vi "Troubleshoot_Apr5_2016.vi"() -> ()   [LabVIEW 2015]
uses:
  <vilib>/Platform/TimedLoop/XDataNode/timing_clust.ctl
  <vilib>/Platform/TimedLoop/XDataNode/nitl_modes.ctl
  <vilib>/Platform/TimedLoop/XDataNode/wakeup.ctl
  <vilib>/FPGAPlugInAG/myRIO-1950/niLvFpga_Open_myRIO-1950.vi
  <vilib>/rvi/interface/common/dynamic/niFpgaDynamicAddResources.vi
  <vilib>/Analysis/3filter.llb/Butterworth Filter (DBL).vi
  <vilib>/Utility/error.llb/Error Cluster From Error Code.vi
  <vilib>/rvi/errors/niLvFpgaAdjustHostInterfaceError.vi
  <vilib>/RVI Host/nirviSupport.llb/nirviErrorClusterFromErrorCode.vi
  <vilib>/rvi/interface/nirviOpenFPGA/nirviOpenFPGA.xnode
  FPGA Bitfiles/Flylaserbox_FPGATarget_FPGAsingleloop_H8b3XToqd60.lvbitx
  FPGA_single_loop.vi
  <vilib>/Platform/TimedLoop/XDataNode/XDataNode.xnode
  <vilib>/rvi/interface/nirviReadWriteControl/nirviReadWriteControl.xnode
  <vilib>/rvi/interface/nirviMethod/nirviMethod.xnode
  <vilib>/Platform/TimedLoop/XDataNode/XDNodeRunTimeDep.lvlib
  <vilib>/rvi/interface/nirviMethod/StockFPGA_InlinedMethodWaitForSingleIRQ.vi
  <vilib>/FPGAPlugInAG/Dynamic/niLvFpga_WaitOnIrq_Dynamic.vi
  NiFpgaLv.dll
  <vilib>/rvi/interface/Simulation/niFpgaSimulationCallBeginRW.vi
  <vilib>/FPGAPlugInAG/Dynamic/niLvFpga_ReadFifo_Dynamic.vi
  <vilib>/rvi/errors/niLvFpgaMergeErrorWithErrorCode.vi
  <vilib>/FPGAPlugInAG/Dynamic/niLvFpga_AcknowledgeIrq_Dynamic.vi
  <vilib>/Analysis/NI_AALBase.lvlib
panel:
  in  "Period":i64
  out "Host loop time":u32=20
  out "Iteration Duration":dbl=4.0 format="%#_6f"
  out "IRQ(s) Asserted":i32
  out "Sensor Loop Time":u32=11
  out "LED loop time":u32=4000
  out "Frame Count":i16=6319
  in  "FPGA Stop":bool
  out "Elements Remaining":u32=3080
  in  "FIFO Timeout setting (ms)":i32=5000
  out "J1":u16[](graph)=[299, 303, 314, 315, 325, 328, 342, 332, 348, 346, 357, 352, 368, 366, 378, 374, 387, 387, 399, 398, 406, 407, 416, 411, 423, 417, 428, 424, 435, 427, 440, 431, 443, 431, 443, 436, 451, 442, 450, 442, 450, 445, 452, 447, 464, 448, 456, 448, 459, 450, 461, 454, 461, 453, 464, 456, 465, 454, 465, 463, 467, 457, 468, 460, 469, 460, 470, 462, 472, 459, 476, 459, 471, 461, 473, 460, 472, 466, 477, 466, 474, 463, 476, 468, 477, 470, 478, 469, 479, 470, 481, 471, 484, 472, 481, 471, 481, 473, 484, 473, 485, 476, 489, 478, 485, 478, 489, 478, 491, 480, 490, 481, 493, 484, 496, 487, 499, 487, 499, 492, 504, 492, 505, 496, 509, 500, 509, 478, 510, 513, 517, 519, 518, 517, 518, 516, 517, 518, 516, 512, 517, 521, 520, 520, 519, 517, 518, 521, 518, 518, 521, 524, 523, 523, 523, 519, 522, 524, 519, 519, 514, 522, 520, 520, 521, 522, 519, 521, 520, 520, 524, 523, 521, 520, 521, 524, 521, 522, 525, 523, 523, 526, 529, 527, 528, 528, 529, 527, 528, 529, 525, 531, 530, 534, 537, 534, 532, 535, 535, 541, 539, 543, 540, 543, 543, 540, 541, 540, 546, 545, 548, 552, 548, 550, 553, 548, 550, 551, 551, 555, 555, 554, 553, 556, 557, 559, 560, 559, 561, 560, 563, 564, 567, 571, 569, 571, 576, 574, 576, 582, 583, 580, 582, 582, 587, 588, 589, 585, 589, 593, 599, 595, 593, 595, 599, 573, 559, 556, 572, 564, 570, 566, 568, 565, 570, 563, 568, 567, 570, 570, 567, 560, 568, 563, 563, 564, 566, 563, 569, 564, 568, 562, 576, 570, 574, 577, 573, 579, 582, 577, 586, 585, 590, 588, 590, 589, 587, 589, 588, 591, 590, 587, 588, 592, 593, 587, 588, 580, 578, 579, 580, 579, 581, 576, 576, 577, 587, 585, 586, 587, 592, 594, 602, 604, 607, 601, 608, 612, 609, 609, 611, 608, 608, 604, 610, 605, 609, 612, 613, 607, 611, 614, 615, 612, 619, 614, 609, 615, 605, 607, 613, 612, 618, 618, 616, 616, 622, 620, 623, 623, 615, 621, 626, 618, 622, 621, 623, 624, 623, 617, 619, 625, 620, 612, 627, 620, 620, 622, 625, 629, 635, 621, 617, 595, 620, 620, 634, 620, 632, 616, 636, 625, 631, 622, 629, 622, 630, 617, 627, 625, 626, 620, 632, 622, 626, 618, 624, 621, 623, 617, 630, 620, 627, 618, 626, 617, 627, 618, 630, 620, 627, 619, 627, 618, 626, 612, 627, 614, 624, 612, 621, 612, 622, 610, 619, 610, 613, 603, 615, 606, 612, 604, 616, 601, 614, 601, 611, 599, 608, 599, 603, 595, 601, 595, 599, 591, 597, 586, 595, 586, 595, 581, 589, 580, 591, 577, 589, 576, 585, 576, 584, 573, 584, 573, 582, 573, 582, 573, 580, 572, 581, 568, 578, 567, 578, 569, 576, 564, 575, 562, 571, 568, 572, 561, 573, 560, 568, 560, 567, 558, 564, 559, 566, 557, 565, 557, 563, 556, 567, 553, 558, 544, 543, 535, 544, 538, 547, 534, 539, 534, 538, 530, 535, 528, 536, 524, 533, 525, 530, 520, 530, 522, 528, 517, 529, 516, 525, 517, 523, 512, 520, 516, 520, 513, 518, 510, 517, 509, 516, 506, 515, 511, 517, 507, 513, 505, 514, 506, 515, 505, 511, 506, 513, 507, 515, 507, 515, 508, 518, 509, 517, 506, 518, 513, 521, 512, 524, 517, 523, 517, 522, 517, 527, 517, 530, 527, 533, 525, 532, 527, 538, 532, 539, 530, 542, 537, 540, 529, 538, 537, 548, 537, 549, 540, 550, 539, 550, 545, 552, 543, 552, 552, 549, 539, 545, 544, 552, 543, 551, 545, 550, 547, 548, 543, 548, 537, 543, 540, 546, 533, 538, 533, 539, 531, 540, 530, 536, 526, 531, 528, 510, 509, 516, 513, 513, 513, 512, 504, 509, 499, 506, 499, 507, 493, 507, 502, 501, 492, 498, 493, 502, 489, 495, 486, 493, 491, 496, 491, 493, 488, 489, 479, 487, 477, 483, 475, 476, 474, 479, 468, 474, 467, 474, 466, 469, 468, 467, 464, 467, 453, 460, 452, 457, 452, 457, 450, 451, 445, 450, 441, 448, 441, 448, 439, 449, 432, 437, 428, 437, 428, 435, 429, 434, 425, 431, 422, 426, 422, 424, 420, 430, 421, 427, 418, 424, 415, 423, 415, 422, 414, 417, 409, 415, 411, 410, 405, 406, 396, 403, 395, 396, 392, 392, 387, 388, 381, 384, 375, 379, 371, 371, 364, 363, 351, 352, 345, 342, 336, 334, 325, 330, 318, 318, 311, 308, 298, 299, 296, 251, 284]
  out "Elements Remaining Real":u32
  out "J4":u16[](graph)=[103, 114, 119, 116, 123, 122, 127, 126, 132, 130, 135, 135, 139, 139, 144, 142, 146, 148, 152, 151, 155, 153, 156, 157, 161, 159, 161, 161, 164, 162, 166, 164, 169, 166, 169, 167, 170, 168, 170, 170, 171, 170, 171, 169, 172, 171, 174, 173, 174, 173, 176, 175, 176, 175, 176, 176, 177, 177, 179, 175, 179, 176, 179, 176, 180, 176, 179, 176, 181, 178, 180, 179, 180, 178, 180, 178, 179, 178, 180, 179, 180, 178, 180, 180, 179, 179, 180, 177, 182, 180, 181, 179, 181, 179, 182, 181, 182, 179, 180, 179, 181, 178, 180, 178, 180, 180, 181, 179, 180, 180, 181, 180, 181, 180, 182, 180, 182, 180, 182, 179, 182, 179, 182, 182, 182, 181, 183, 179, 185, 185, 188, 186, 188, 186, 187, 184, 187, 185, 186, 185, 186, 184, 185, 184, 187, 185, 186, 185, 188, 185, 187, 186, 188, 185, 188, 185, 186, 187, 187, 185, 188, 185, 187, 184, 188, 186, 187, 185, 188, 185, 187, 185, 187, 184, 185, 186, 187, 185, 187, 185, 188, 186, 189, 188, 190, 187, 189, 188, 190, 187, 191, 190, 194, 189, 192, 191, 193, 192, 194, 194, 197, 195, 198, 196, 197, 196, 199, 196, 200, 199, 201, 200, 203, 202, 205, 203, 204, 204, 207, 202, 206, 205, 205, 203, 206, 201, 204, 202, 205, 202, 204, 202, 203, 201, 202, 200, 202, 201, 203, 200, 203, 200, 200, 200, 201, 198, 201, 200, 201, 198, 201, 200, 201, 199, 201, 201, 190, 188, 191, 188, 192, 189, 191, 188, 191, 188, 191, 189, 189, 189, 190, 189, 189, 186, 190, 188, 190, 187, 189, 188, 190, 187, 189, 187, 190, 186, 189, 187, 190, 186, 188, 185, 190, 186, 189, 185, 189, 186, 189, 186, 190, 187, 190, 187, 190, 187, 194, 188, 193, 189, 191, 189, 192, 188, 192, 188, 192, 189, 190, 187, 191, 187, 190, 189, 190, 187, 191, 188, 191, 188, 191, 188, 192, 187, 190, 189, 191, 188, 191, 188, 192, 189, 194, 189, 192, 188, 191, 187, 192, 187, 191, 188, 190, 186, 191, 186, 188, 184, 189, 183, 187, 183, 187, 183, 187, 182, 186, 182, 187, 182, 186, 183, 185, 183, 188, 184, 189, 184, 188, 184, 188, 183, 186, 182, 187, 186, 190, 188, 189, 189, 190, 188, 188, 186, 189, 188, 189, 187, 188, 186, 188, 186, 187, 185, 187, 186, 187, 188, 189, 189, 191, 188, 190, 189, 189, 189, 188, 186, 189, 188, 187, 186, 188, 187, 187, 187, 186, 187, 187, 186, 186, 186, 186, 186, 188, 184, 185, 183, 186, 184, 186, 184, 184, 185, 185, 184, 186, 184, 183, 182, 182, 182, 185, 182, 183, 183, 184, 182, 183, 183, 182, 181, 183, 180, 181, 180, 180, 180, 180, 179, 180, 178, 180, 178, 179, 178, 178, 178, 180, 180, 181, 177, 179, 180, 179, 178, 179, 177, 179, 178, 178, 177, 176, 175, 178, 176, 177, 175, 178, 175, 176, 175, 176, 176, 176, 173, 174, 174, 176, 173, 173, 170, 178, 176, 180, 177, 179, 176, 179, 177, 178, 174, 179, 173, 178, 175, 177, 173, 178, 174, 176, 174, 176, 173, 176, 172, 176, 174, 176, 172, 175, 170, 174, 171, 173, 169, 171, 168, 172, 168, 170, 169, 170, 166, 169, 167, 170, 166, 168, 165, 167, 166, 167, 166, 167, 164, 166, 164, 166, 164, 165, 163, 166, 164, 167, 163, 168, 162, 164, 162, 166, 163, 167, 163, 167, 163, 166, 164, 167, 163, 167, 164, 167, 164, 168, 165, 168, 163, 168, 166, 167, 165, 169, 166, 169, 165, 168, 165, 168, 165, 168, 164, 167, 165, 168, 165, 168, 166, 167, 165, 168, 165, 167, 165, 168, 164, 165, 164, 167, 164, 167, 163, 165, 162, 167, 162, 165, 162, 166, 163, 173, 166, 170, 167, 171, 167, 172, 169, 171, 167, 172, 168, 173, 170, 173, 168, 172, 170, 173, 170, 172, 171, 174, 170, 175, 171, 175, 171, 173, 172, 174, 172, 175, 170, 175, 172, 176, 172, 176, 172, 176, 170, 174, 172, 174, 171, 174, 171, 175, 171, 173, 171, 175, 172, 174, 171, 173, 170, 175, 171, 175, 172, 175, 172, 175, 172, 174, 171, 175, 170, 175, 171, 175, 171, 176, 171, 173, 173, 172, 170, 173, 171, 173, 169, 173, 171, 173, 169, 172, 168, 171, 168, 170, 166, 170, 165, 168, 164, 166, 161, 164, 160, 162, 158, 159, 156, 156, 153, 155, 152, 152, 148, 148, 144, 145, 139, 141, 136, 137, 132, 133, 127, 128, 122, 124, 118, 120, 115, 28, 119]
  out "J8":u16[](graph)=[148, 165, 179, 176, 192, 190, 205, 200, 215, 212, 228, 224, 240, 236, 249, 243, 258, 256, 266, 263, 273, 268, 282, 276, 288, 282, 293, 287, 299, 289, 302, 295, 305, 298, 306, 300, 308, 302, 313, 302, 310, 304, 314, 305, 312, 306, 315, 306, 314, 305, 315, 305, 315, 304, 313, 303, 315, 305, 315, 304, 316, 307, 315, 306, 318, 308, 318, 308, 318, 310, 318, 309, 320, 311, 320, 313, 323, 316, 323, 314, 326, 316, 326, 317, 329, 321, 330, 319, 329, 321, 330, 321, 329, 319, 329, 320, 329, 319, 327, 320, 329, 318, 328, 320, 328, 320, 328, 318, 327, 319, 327, 317, 328, 318, 327, 317, 323, 315, 326, 316, 327, 317, 329, 321, 329, 320, 326, 319, 321, 320, 327, 324, 330, 324, 330, 328, 335, 329, 336, 333, 339, 336, 339, 337, 343, 336, 344, 339, 346, 340, 346, 344, 350, 345, 351, 348, 354, 348, 355, 351, 356, 351, 359, 352, 359, 354, 360, 357, 363, 359, 364, 359, 367, 362, 367, 363, 369, 362, 369, 361, 368, 362, 367, 362, 367, 360, 365, 358, 365, 359, 363, 359, 365, 358, 365, 360, 366, 358, 367, 362, 368, 360, 369, 364, 368, 365, 372, 368, 373, 369, 377, 373, 378, 372, 380, 376, 382, 376, 384, 381, 385, 379, 387, 384, 388, 382, 390, 382, 390, 385, 390, 386, 391, 387, 392, 386, 393, 388, 395, 388, 396, 389, 396, 392, 396, 393, 398, 392, 400, 390, 397, 393, 400, 392, 392, 386, 407, 408, 410, 409, 409, 405, 409, 408, 409, 405, 410, 408, 411, 409, 412, 408, 410, 411, 413, 411, 415, 414, 416, 413, 418, 416, 418, 414, 416, 414, 415, 411, 413, 412, 414, 410, 412, 411, 414, 409, 410, 408, 411, 405, 410, 405, 407, 405, 404, 402, 405, 401, 402, 398, 401, 398, 399, 394, 398, 393, 394, 390, 392, 390, 392, 388, 392, 389, 389, 388, 391, 388, 389, 388, 390, 387, 388, 384, 390, 388, 388, 386, 389, 385, 388, 385, 387, 383, 389, 386, 389, 386, 391, 390, 389, 391, 392, 391, 394, 392, 397, 394, 396, 396, 398, 396, 401, 399, 402, 401, 404, 402, 405, 402, 406, 402, 406, 405, 407, 406, 409, 407, 409, 407, 408, 409, 413, 404, 400, 402, 403, 401, 396, 396, 393, 393, 390, 390, 390, 389, 385, 387, 387, 388, 387, 387, 387, 387, 386, 388, 385, 387, 385, 387, 387, 386, 385, 388, 385, 386, 385, 384, 386, 388, 387, 387, 386, 389, 389, 387, 387, 390, 390, 391, 392, 394, 394, 394, 393, 395, 394, 395, 394, 397, 396, 398, 396, 398, 398, 395, 396, 398, 398, 398, 397, 396, 395, 395, 393, 395, 393, 395, 391, 393, 393, 393, 391, 390, 390, 390, 387, 387, 385, 385, 382, 382, 381, 380, 379, 380, 378, 379, 376, 377, 376, 376, 374, 373, 375, 375, 373, 373, 373, 371, 372, 373, 369, 369, 371, 371, 368, 370, 369, 370, 369, 369, 369, 369, 368, 369, 369, 370, 368, 370, 372, 375, 350, 349, 354, 350, 354, 352, 353, 352, 355, 353, 356, 354, 357, 353, 357, 354, 358, 353, 358, 355, 358, 355, 357, 353, 358, 354, 356, 354, 359, 353, 357, 355, 357, 353, 357, 354, 358, 353, 358, 356, 359, 354, 358, 356, 359, 356, 358, 355, 359, 357, 361, 355, 360, 356, 358, 356, 360, 356, 360, 356, 359, 358, 361, 358, 361, 361, 363, 360, 365, 363, 368, 363, 365, 363, 367, 363, 367, 363, 366, 363, 366, 363, 367, 361, 362, 359, 359, 356, 357, 353, 355, 351, 354, 351, 355, 350, 353, 349, 353, 352, 353, 349, 352, 348, 351, 346, 350, 346, 347, 342, 348, 344, 346, 341, 348, 344, 345, 342, 345, 341, 345, 342, 342, 338, 342, 337, 337, 333, 334, 342, 335, 340, 337, 341, 337, 342, 339, 341, 335, 339, 335, 340, 334, 339, 334, 339, 331, 336, 332, 334, 331, 336, 330, 335, 331, 335, 326, 334, 329, 333, 328, 333, 328, 333, 327, 334, 328, 333, 328, 334, 329, 333, 328, 332, 327, 331, 324, 330, 327, 331, 326, 331, 325, 329, 324, 330, 326, 327, 326, 329, 325, 330, 325, 329, 325, 329, 325, 330, 323, 329, 325, 327, 323, 328, 325, 325, 321, 324, 318, 324, 317, 322, 318, 315, 303, 309, 310, 312, 309, 311, 306, 309, 304, 305, 301, 301, 297, 298, 293, 293, 285, 286, 281, 283, 276, 275, 269, 271, 262, 261, 254, 253, 244, 243, 236, 233, 226, 220, 214, 211, 202, 200, 193, 189, 180, 178, 125, 198]
  out "J5":u16[](graph)=[173, 183, 200, 196, 214, 209, 228, 224, 240, 234, 253, 246, 263, 257, 274, 266, 284, 278, 291, 283, 299, 289, 307, 296, 312, 302, 318, 307, 320, 309, 323, 312, 324, 313, 324, 315, 326, 315, 327, 319, 329, 318, 331, 318, 332, 321, 334, 323, 338, 324, 338, 327, 339, 327, 340, 328, 344, 331, 343, 332, 345, 334, 347, 336, 350, 339, 351, 339, 352, 340, 354, 343, 357, 345, 359, 348, 360, 350, 363, 351, 364, 352, 365, 354, 367, 355, 367, 358, 370, 358, 371, 358, 369, 359, 371, 361, 373, 360, 372, 360, 371, 359, 372, 360, 372, 360, 371, 359, 371, 359, 369, 358, 371, 358, 369, 354, 367, 357, 367, 354, 368, 354, 367, 354, 364, 353, 362, 342, 355, 345, 350, 344, 349, 344, 347, 344, 348, 340, 347, 340, 346, 341, 348, 341, 346, 339, 345, 339, 345, 338, 343, 337, 344, 338, 342, 338, 341, 338, 344, 339, 344, 338, 342, 339, 344, 339, 344, 340, 346, 340, 347, 341, 347, 343, 349, 344, 350, 346, 352, 347, 353, 350, 357, 352, 357, 353, 360, 358, 364, 360, 367, 364, 373, 367, 372, 372, 379, 375, 380, 378, 386, 384, 391, 387, 394, 392, 399, 397, 406, 401, 409, 405, 412, 408, 415, 412, 419, 417, 424, 420, 426, 421, 428, 426, 432, 429, 435, 431, 438, 434, 440, 438, 442, 441, 446, 441, 449, 444, 453, 450, 457, 455, 461, 457, 463, 463, 469, 466, 474, 468, 475, 472, 478, 474, 479, 471, 476, 462, 464, 462, 465, 463, 465, 462, 468, 461, 465, 461, 463, 459, 463, 459, 461, 457, 458, 454, 457, 452, 453, 451, 452, 446, 448, 444, 448, 442, 445, 440, 444, 437, 441, 436, 439, 436, 439, 435, 439, 434, 438, 436, 439, 435, 438, 435, 440, 436, 441, 440, 444, 440, 445, 444, 447, 445, 451, 448, 449, 446, 451, 448, 454, 449, 456, 452, 455, 454, 459, 457, 460, 458, 463, 460, 462, 458, 463, 460, 465, 464, 468, 463, 468, 466, 468, 466, 468, 465, 471, 468, 469, 464, 466, 464, 467, 462, 466, 462, 464, 461, 462, 459, 460, 457, 459, 459, 460, 454, 456, 452, 455, 452, 454, 448, 451, 446, 451, 443, 447, 443, 444, 440, 439, 436, 438, 437, 441, 438, 438, 434, 437, 437, 438, 437, 437, 438, 439, 437, 439, 437, 436, 435, 440, 437, 437, 435, 438, 434, 434, 436, 436, 436, 437, 434, 434, 433, 434, 432, 432, 432, 432, 432, 434, 431, 431, 431, 429, 430, 430, 429, 429, 427, 428, 425, 427, 425, 426, 425, 424, 424, 422, 419, 422, 419, 421, 417, 420, 416, 418, 416, 418, 412, 413, 411, 413, 411, 410, 409, 409, 407, 408, 405, 405, 404, 403, 403, 403, 401, 402, 400, 400, 399, 399, 398, 400, 397, 398, 397, 397, 395, 396, 396, 397, 395, 395, 394, 394, 392, 393, 392, 393, 390, 390, 389, 391, 389, 389, 387, 388, 387, 389, 385, 386, 384, 385, 382, 384, 380, 380, 381, 380, 376, 376, 381, 402, 382, 392, 379, 390, 381, 391, 382, 393, 383, 392, 382, 391, 384, 392, 385, 393, 385, 393, 383, 392, 383, 391, 381, 392, 384, 390, 380, 390, 380, 391, 381, 392, 381, 389, 379, 389, 379, 390, 378, 388, 380, 389, 378, 386, 378, 388, 378, 387, 376, 389, 379, 386, 377, 388, 379, 388, 378, 389, 380, 391, 380, 390, 381, 391, 382, 392, 383, 393, 384, 394, 384, 394, 383, 394, 386, 396, 384, 392, 384, 394, 383, 394, 384, 392, 381, 389, 379, 390, 379, 386, 377, 386, 372, 383, 372, 381, 371, 379, 369, 377, 367, 375, 366, 373, 363, 373, 363, 371, 361, 369, 358, 367, 356, 365, 356, 363, 353, 361, 352, 359, 349, 358, 347, 359, 349, 354, 352, 355, 349, 352, 348, 352, 350, 351, 350, 351, 349, 353, 351, 351, 347, 349, 345, 351, 345, 348, 344, 349, 344, 345, 344, 347, 342, 344, 341, 344, 341, 343, 341, 345, 341, 345, 340, 342, 339, 340, 343, 341, 339, 340, 338, 339, 338, 339, 337, 338, 336, 338, 336, 337, 337, 340, 337, 338, 339, 338, 338, 339, 336, 337, 336, 338, 335, 337, 334, 337, 334, 336, 333, 337, 333, 333, 334, 335, 332, 333, 332, 332, 329, 329, 327, 330, 326, 326, 324, 325, 322, 322, 319, 321, 318, 320, 316, 317, 313, 314, 309, 311, 305, 307, 302, 301, 297, 295, 289, 289, 284, 283, 277, 276, 268, 267, 261, 257, 248, 244, 237, 234, 227, 223, 215, 212, 202, 200, 195, 172, 227]
  out "Finished Late? [i-1]":bool
  out "Has timed loop ever been late?":bool
  in  "Threshold for noise filter":dbl=8.0
  out "Fly real-time location/center mass":dbl(graph)=731.3095378093176
  in  "Fly presence? J1":bool=TRUE
  in  "Threshhold position filter J1":i32=25
  out "Fly real-time location J1":dbl(graph)=731.3095378093176
  in  "Threshold for noise filter J4":dbl=7.0
  in  "Threshhold position filter J4":i32=25
  in  "Fly presence? J4":bool=TRUE
  out "Fly real-time location J4":dbl(graph)=203.38593568844155
  in  "Threshold for noise filter J5":dbl=5.0
  in  "Threshhold position filter J5":i32=25
  out "Fly real-time location J5":dbl(graph)=118.45001929078613
  in  "Fly presence? J5":bool=TRUE
  in  "Threshold for noise filter J8":dbl=5.0
  in  "Threshhold position filter J8":i32=25
  in  "Fly presence? J8":bool=TRUE
  out "Fly real-time location J8":dbl(graph)=209.002598036444
  out "Noise check J1":dbl[](graph)=[0.0, 0.0, 0.0, 0.0, 0.0, 0.0, 0.0, 0.0, 0.0, 0.0, 0.0, 0.0, 0.0, 0.0, 0.0, 0.0, 0.0, 0.0, 0.0, 0.0, 0.0, 0.0, 0.0, 0.0, 0.0, 0.0, 0.0, 0.0, 0.0, 0.0, 0.0, 0.0, 0.0, 0.0, 0.0, 0.0, 0.0, 0.0, 0.0, 0.0, 0.0, 0.0, 0.0, 0.0, 0.0, 0.0, 0.0, 0.0, 0.0, 0.0, 0.0, 0.0, 0.0, 0.0, 0.0, 0.0, 0.0, 0.0, 0.0, 0.0, 0.0, 0.0, 0.0, 0.0, 0.0, 0.0, 0.0, 0.0, 0.0, 0.0, 0.0, 0.0, 0.0, 0.0, 0.0, 0.0, 0.0, 0.0, 0.0, 0.0, 0.0, 0.0, 0.0, 0.0, 0.0, 0.0, 0.0, 0.0, 0.0, 0.0, 0.0, 0.0, 0.0, 0.0, 0.0, 0.0, 0.0, 0.0, 0.0, 0.0, 0.0, 0.0, 0.0, 0.0, 0.0, 0.0, 0.0, 0.0, 0.0, 0.0, 0.0, 0.0, 0.0, 0.0, 0.0, 0.0, 0.0, 0.0, 0.0, 0.0, 0.0, 0.0, 0.0, 0.0, 0.0, 0.0, 0.0, 0.0, 0.0, 0.0, 0.0, 0.0, 0.0, 0.0, 0.0, 0.0, 0.0, 0.0, 0.0, 0.0, 0.0, 0.0, 0.0, 0.0, 0.0, 0.0, 0.0, 0.0, 0.0, 0.0, 0.0, 0.0, 0.0, 0.0, 0.0, 0.0, 0.0, 0.0, 0.0, 0.0, 0.0, 0.0, 0.0, 0.0, 0.0, 0.0, 0.0, 0.0, 0.0, 0.0, 0.0, 0.0, 0.0, 0.0, 0.0, 0.0, 0.0, 0.0, 0.0, 0.0, 0.0, 0.0, 0.0, 0.0, 0.0, 0.0, 0.0, 0.0, 0.0, 0.0, 0.0, 0.0, 0.0, 0.0, 0.0, 0.0, 0.0, 0.0, 0.0, 0.0, 0.0, 0.0, 0.0, 0.0, 0.0, 0.0, 0.0, 0.0, 0.0, 0.0, 0.0, 0.0, 0.0, 0.0, 0.0, 0.0, 0.0, 0.0, 0.0, 0.0, 0.0, 0.0, 0.0, 0.0, 0.0, 0.0, 0.0, 0.0, 0.0, 0.0, 0.0, 0.0, 0.0, 0.0, 0.0, 0.0, 0.0, 0.0, 0.0, 0.0, 0.0, 0.0, 0.0, 0.0, 0.0, 0.0, 0.0, 0.0, 0.0, 0.0, 0.0, 0.0, 0.0, 0.0, 0.0, 0.0, 0.0, 0.0, 0.0, 0.0, 0.0, 0.0, 0.0, 0.0, 0.0, 0.0, 0.0, 0.0, 0.0, 0.0, 0.0, 0.0, 0.0, 0.0, 0.0, 0.0, 0.0, 0.0, 0.0, 0.0, 0.0, 0.0, 0.0, 0.0, 0.0, 0.0, 0.0, 0.0, 0.0, 0.0, 0.0, 0.0, 0.0, 0.0, 0.0, 0.0, 0.0, 0.0, 0.0, 0.0, 0.0, 0.0, 0.0, 0.0, 0.0, 0.0, 0.0, 0.0, 0.0, 0.0, 0.0, 0.0, 0.0, 0.0, 0.0, 0.0, 0.0, 0.0, 0.0, 0.0, 0.0, 0.0, 0.0, 0.0, 0.0, 0.0, 0.0, 0.0, 0.0, 0.0, 0.0, 0.0, 0.0, 0.0, 0.0, 0.0, 0.0, 0.0, 0.0, 0.0, 0.0, 0.0, 0.0, 0.0, 0.0, 0.0, 0.0, 0.0, 0.0, 0.0, 0.0, 0.0, 0.0, 0.0, 0.0, 0.0, 0.0, 0.0, 0.0, 0.0, 0.0, 0.0, 0.0, 0.0, 0.0, 0.0, 0.0, 0.0, 0.0, 0.0, 0.0, 0.0, 0.0, 0.0, 0.0, 0.0, 0.0, 0.0, 0.0, 0.0, 0.0, 0.0, 0.0, 0.0, 0.0, 0.0, 0.0, 0.0, 0.0, 0.0, 0.0, 0.0, 0.0, 0.0, 0.0, 0.0, 0.0, 0.0, 0.0, 0.0, 0.0, 0.0, 0.0, 0.0, 0.0, 0.0, 0.0, 0.0, 0.0, 0.0, 0.0, 0.0, 0.0, 0.0, 0.0, 0.0, 0.0, 0.0, 0.0, 0.0, 0.0, 0.0, 0.0, 0.0, 0.0, 0.0, 0.0, 0.0, 0.0, 0.0, 0.0, 0.0, 0.0, 0.0, 0.0, 0.0, 0.0, 0.0, 0.0, 0.0, 0.0, 0.0, 0.0, 0.0, 0.0, 0.0, 0.0, 0.0, 0.0, 0.0, 0.0, 0.0, 0.0, 0.0, 0.0, 0.0, 0.0, 0.0, 0.0, 0.0, 0.0, 0.0, 0.0, 0.0, 0.0, 0.0, 0.0, 0.0, 0.0, 0.0, 0.0, 0.0, 0.0, 0.0, 0.0, 0.0, 0.0, 0.0, 0.0, 0.0, 0.0, 0.0, 0.0, 0.0, 0.0, 0.0, 0.0, 0.0, 0.0, 0.0, 0.0, 0.0, 0.0, 0.0, 0.0, 0.0, 0.0, 0.0, 0.0, 0.0, 0.0, 0.0, 0.0, 0.0, 0.0, 0.0, 0.0, 0.0, 0.0, 0.0, 0.0, 0.0, 0.0, 0.0, 0.0, 0.0, 0.0, 0.0, 0.0, 0.0, 0.0, 0.0, 0.0, 0.0, 0.0, 0.0, 0.0, 0.0, 0.0, 0.0, 0.0, 0.0, 0.0, 0.0, 0.0, 0.0, 0.0, 0.0, 0.0, 0.0, 0.0, 0.0, 0.0, 0.0, 0.0, 0.0, 0.0, 0.0, 0.0, 0.0, 0.0, 0.0, 0.0, 0.0, 0.0, 0.0, 0.0, 0.0, 0.0, 0.0, 0.0, 0.0, 0.0, 0.0, 0.0, 0.0, 0.0, 0.0, 0.0, 0.0, 0.0, 0.0, 0.0, 0.0, 0.0, 0.0, 0.0, 0.0, 0.0, 0.0, 0.0, 0.0, 0.0, 0.0, 0.0, 0.0, 0.0, 0.0, 0.0, 0.0, 0.0, 0.0, 0.0, 0.0, 0.0, 0.0, 0.0, 0.0, 0.0, 0.0, 0.0, 0.0, 0.0, 0.0, 0.0, 0.0, 0.0, 0.0, 0.0, 0.0, 0.0, 0.0, 0.0, 0.0, 0.0, 0.0, 0.0, 0.0, 0.0, 0.0, 0.0, 0.0, 0.0, 0.0, 0.0, 0.0, 0.0, 0.0, 0.0, 0.0, 0.0, 0.0, 0.0, 0.0, 0.0, 0.0, 0.0, 0.0, 0.0, 0.0, 0.0, 0.0, 0.0, 0.0, 0.0, 0.0, 0.0, 0.0, 0.0, 0.0, 0.0, 0.0, 0.0, 0.0, 0.0, 0.0, 0.0, 0.0, 0.0, 0.0, 0.0, 0.0, 0.0, 0.0, 0.0, 0.0, 0.0, 0.0, 0.0, 0.0, 0.0, 0.0, 0.0, 0.0, 0.0, 0.0, 0.0, 0.0, 0.0, 0.0, 0.0, 0.0, 0.0, 0.0, 0.0, 0.0, 0.0, 0.0, 0.0, 0.0, 0.0, 0.0, 0.0, 0.0, 0.0, 0.0, 0.0, 0.0, 0.0, 0.0, 0.0, 0.0, 0.0, 0.0, 0.0, 0.0, 0.0, 0.0, 0.0, 0.0, 0.0, 0.0, 0.0, 0.002630031854768592, 0.02647244479643197, 0.07238343896731143, 0.0945645708112122, 0.07323461692650168, 0.0403804808476501, 0.05121951335433386, 0.1762106489274184, 0.44006181658327786, 0.7845113623785474, 1.119997669332286, 1.3668328869065776, 1.4775687137089684, 1.4816747529196042, 1.4845963350311595, 1.5954761742667545, 1.8331785662226308, 2.090278012312389, 2.2184400479496444, 2.1448325104345916, 1.9046852618093164, 1.611675881479425, 1.3951054047298297, 1.310250193006133, 1.3163036215716177, 1.3380381305237252, 1.2993463614109941, 1.1409959811952943, 0.8726900095644392, 0.5720582464254442, 0.3083972063095004, 0.1147690458320547, 0.00540622533437389, -0.033159310484607185, -0.033064972848972515, -0.02012085186680765, -0.007948463448035415, -0.0007869325832231132, 0.0019075606614335245, 0.002060776300040158, 0.0013070649745447168, 0.0005453872425892686, 7.850769862843349e-05, -0.00010777797942906934, -0.00012778328636531668, -8.45492446052674e-05, -3.7119363484340684e-05, -6.8133899757183335e-06, 5.949395488515054e-06, 7.88027385042564e-06, 5.4464616068189726e-06, 2.508215297396619e-06, 5.492808583469846e-07, -3.1820480618137934e-07, -4.830999877916673e-07]
  out "Noise check J4":dbl[](graph)
  out "Noise check J5":dbl[](graph)=[0.0, 0.0, 0.0, 0.0, 0.0, 0.0, 0.0, 0.0, 0.0, 0.0, 0.0, 0.0, 0.0, 0.0, 0.0, 0.0, 0.0, 0.0, 0.0, 0.0, 0.0, 0.0, 0.0, 0.0, 0.0, 0.0, 0.0, 0.0, 0.0, 0.0, 0.0, 0.0, 0.0, 0.0, 0.0, 0.0, 0.0, 0.0, 0.0, 0.0, 0.0, 0.0, 0.0, 0.0, 0.0, 0.0, 0.0, 0.0, 0.0, 0.0, 0.0, 0.0, 0.0, 0.0, 0.0, 0.0, 0.0, 0.0, 0.0, 0.0, 0.0, 0.0, 0.0, 0.0, 0.0, 0.0, 0.0, 0.0, 0.0, 0.0, 0.0, 0.0, 0.0, 0.0, 0.0, 0.0, 0.0, 0.0, 0.012054538365298214, 0.08251007933289906, 0.2697925233234689, 0.5818524655936519, 0.9729636503034512, 1.3844748873925616, 1.7368973639426482, 1.9514883967448342, 2.049795713035472, 2.147680935919143, 2.3188998494047826, 2.5331530921105125, 2.708069472184627, 2.8118388391573657, 2.9368447973981366, 3.211657108218735, 3.6431393080511585, 4.115369018049598, 4.513477004341131, 4.788356388610584, 4.94484597379937, 5.027249271232393, 5.089663667941105, 5.167005021431631, 5.29495778292663, 5.524154011291435, 5.879990611460722, 6.317736798856551, 6.728055846578749, 6.994230662169988, 7.050570723594823, 6.91770548084906, 6.7126808158556095, 6.591977061099051, 6.647863503971012, 6.837387129399459, 7.006122980790215, 7.02845268511157, 6.943869825354531, 6.8908804792545695, 6.913056904386163, 6.940669455926634, 6.926706265783624, 6.891548364808854, 6.879976507396142, 6.9238783794600405, 7.014599560394951, 7.097802219395696, 7.099555418502421, 6.98268555249647, 6.792270609676624, 6.6049691690102215, 6.434305425951933, 6.237108330326169, 6.01320772445422, 5.836092870646612, 5.7530536936199, 5.715991836295783, 5.633548975996455, 5.4546187281227265, 5.208524422197506, 4.96463488228587, 4.769010412200817, 4.626611813331992, 4.494516771543445, 4.31103555561957, 4.054161846296417, 3.746066456881264, 3.4211563867039594, 3.099985192886244, 2.7794014976662895, 2.44637263169793, 2.0912750035506713, 1.7110175602290862, 1.3259640476500372, 0.9785330169390857, 0.6675468418740619, 0.3718185768752308, 0.13600990134847535, 0.00429183911095006, -0.04129024906400588, -0.04035943318370341, -0.024287822164054097, -0.009445633942039625, -0.0008094883626780184, 0.0023853516999582454, 0.002518760604299784, 0.0015795930379951223, 0.0006496677301419525, 8.598159733688785e-05, -0.0001354916826684314, -0.0001564033159245941, -0.00010229456616431273, -4.430980324289726e-05, -7.677494406688178e-06, 7.531523270977754e-06, 9.659953038992932e-06, 6.5969833094280795e-06, 2.9997111649637766e-06, 6.291603719864854e-07, -4.067256343405995e-07, -5.931847294950123e-07, -4.2368471484944137e-07, -2.017255367751674e-07, -4.896042170647565e-08, 2.108151732718652e-08, 3.6195985715165595e-08, 2.709873015883781e-08, 1.3483599237422958e-08, 3.6795492211654384e-09, -1.025420804479972e-09, -2.1932924129452164e-09, -1.7260489829314328e-09, -8.962371163395401e-10, -2.696307957092095e-10, 4.4535353362904505e-11, 1.3186526572366835e-10, 1.0947864700726096e-10, 5.92623696840606e-11, 1.9380215627957422e-11, -1.4822807061719387e-12, -7.857579527927355e-12, -6.914103455156049e-12, -3.89948607597912e-12, -1.371769578237791e-12, 6.511930663237629e-15, 4.633960331867196e-13, 4.347233263672884e-13, 2.553957382901364e-13, 9.58816357857041e-14, 5.266160377061325e-15, -2.6995561643986745e-14, -2.720704639289042e-14, -1.665252878596416e-14, -6.631139240315776e-15, -7.0105510310460695e-16, 1.5494186569176565e-15, 1.6944909533061055e-15, 1.0811085060167869e-15, 4.54448556635201e-16, 6.808870612399017e-17, -8.728820444841173e-17, -1.0499234375208962e-16, -6.989166283689154e-17, -3.0897043736463205e-17, -5.832791247263445e-18, 4.7998062532403726e-18, 6.469564482484962e-18, 4.499628471438213e-18, 2.0857689124703708e-18, 4.666056321817816e-19, -2.5533629528269204e-19, -3.9626857856385e-19, -2.8849350033730597e-19, -1.3990475436771997e-19, -3.573896726576872e-20, 1.293989664760119e-20, 2.4112840645085403e-20, 1.8420505295880255e-20, 9.329405395104378e-21, 2.655679327128802e-21, -6.06003317208522e-22, -1.456571849069185e-21, -1.1712680032801579e-21, -6.187581139185739e-22, -1.9294807659464302e-22, 2.433951347022674e-23, 8.726353889898586e-23, 7.415968231766969e-23, 4.0830572710290474e-23, 1.377553901834581e-23, -6.2248816426723375e-25, -5.178733808997571e-24, -4.675061004313882e-24, -2.681445181815658e-24, -9.697370938178341e-25, -2.046183940374795e-26, 3.0395409074202434e-25, 2.93391278112018e-25, 1.7529391947798681e-25, 6.747159951419807e-26, 5.181527579327607e-27, -1.7605342120402465e-26, -1.8325651591036842e-26, -1.1409142639444767e-26, -4.648092306822356e-27, -5.792159064985569e-28, 1.0032741085991282e-27, 1.138967869605295e-27, 7.394045026689562e-28, 3.1746129396768222e-28, 5.283721074875335e-29, -5.600503129665911e-29, -7.04144534634944e-29, -4.7719039617888896e-29, -2.1518457519526855e-29, -4.381449771013153e-30, 3.041948713826757e-30, 4.328460008429178e-30, 3.066928327464483e-30, 1.4487077542079428e-30, 3.435453267891325e-31, -1.590049444459223e-31, -2.6442640820958e-31, -1.963019603444207e-31, -9.693312702314344e-32, -2.5955441804768686e-32, 7.840017129254836e-33, 1.6043452970542605e-32, 1.251257347573923e-32, 6.449149749539311e-33, 1.9094588691359505e-33, -3.4946149682933526e-34, -9.659617486074822e-34, -7.942303047997757e-34, -4.268202629278789e-34, -1.3766656808557905e-34, 1.2480135861303e-35, 5.765524095873537e-35, 5.01978371833872e-35, 2.8108561111449943e-35, 9.768393167274569e-36, -1.5979097064840415e-37, -3.406783427648679e-36, -3.158682561416305e-36, -1.8424400025079897e-36, -6.8417490579824315e-37, -3.08996197074768e-38, 1.9892586109109132e-37, 1.97848973677004e-37, 1.2022518088671383e-37, 4.739972967349818e-38, 4.6138334091484117e-39, -1.1449946036667541e-38, -1.2333057118713003e-38, -7.811069082981466e-39, -3.253327516286039e-39, -4.6357690325503895e-40, 6.473780095712158e-40, 7.648794751634878e-40, 5.053426150476074e-40, 2.2148176150911223e-40, 4.0367468947110693e-41, -3.576843912725162e-41, -4.717863079482069e-41, -3.25576266404017e-41, -1.496941450408354e-41, -3.260757128172403e-42, 1.9155335318504096e-42, 2.892901376006323e-42, 2.0889423964204834e-42, 1.0051733200205593e-42, 2.5137236233228282e-43, -9.806163732946778e-44, -1.7624418575065763e-43, -1.3347739940883268e-43, -6.709563709262192e-44, -1.8765906832021888e-44, 4.672545729490458e-45, 1.0660620638309889e-44, 8.493414283511421e-45, 4.454127567626845e-45, 1.3682536486147045e-45, -1.947072781173578e-46, -6.396563318091131e-46, -5.3817134709572885e-46, -2.9417403469254757e-46, -9.795949067489972e-47, 5.70091804711327e-48, 3.8028040638436656e-47, 3.395287453186378e-47, 1.9335063550196973e-47, 6.911647890734894e-48, 7.134294021746332e-50, -2.2366198611548918e-48, -2.1324864077513384e-48, -1.2649875125605185e-48, -4.818128617466808e-49, -3.259501821845982e-50, 1.2987340936199763e-49, 1.3331083068039984e-49, 8.239552005229725e-50, 3.3246297731028743e-50, 3.8797367491773775e-51, -7.424248357593614e-51, -8.292894061549167e-51, -5.343866049579547e-51, -2.2739472080306295e-51, -3.6260930461838345e-52, 4.1611107172087994e-52, 5.1318304892697584e-52, 3.451299279413764e-52, 1.5433060027470366e-52, 3.046097601798571e-53, -2.27246498197299e-53, -3.1578663989489454e-53, -2.219776665712926e-53, -1.0402033777440495e-53, -2.4078759438364993e-54, 1.1971773816231694e-54, 1.9313349743840303e-54, 1.4218209489652026e-54, 6.967273214005052e-55, 1.8294050181191415e-55, -5.976448128700266e-56, -1.1732666059348616e-55, -9.069514266383446e-56, -4.639931366654287e-56, -1.351397822674065e-56, 2.725337028933403e-57, 7.074131801150358e-57, 5.761109747156628e-57, 3.073582425449035e-57, 9.774313850422019e-58, -1.0299632780581152e-58, -4.229163307858031e-58, -3.6439723122896195e-58, -2.0258489406820065e-58, -6.95331260724567e-59, 1.9718380721558834e-60, 2.503677545378321e-59, 2.294761891250138e-59, 1.3289630775558111e-59, 4.880377750316307e-60, 1.7138734414810517e-61, -1.4652070457631984e-60, -1.438539565251322e-60, -8.678657602047437e-61, -3.387184971834156e-61, -3.0058274960698244e-62, 8.456695232049919e-62, 8.974991225370526e-62, 5.642804464715705e-62, 2.3284233274234247e-62, 3.1432374415349554e-63, -4.797938411692989e-63, -5.571285529343017e-63, -3.6533455664022435e-63, -1.587312055580106e-63, -2.7875030234571983e-64, 2.6629571313142356e-64, 3.439827735234227e-64, 2.355448313158835e-64, 1.0741287215472925e-64, 2.2754883277815795e-65, -1.4350781023773857e-65, -2.1115007195583554e-65, -1.5123826022475209e-65, -7.220544185442533e-66, -1.766319002352943e-66, 7.415465360776138e-67, 1.287909779752148e-66, 9.670708063997506e-67, 4.824598402063589e-67, 1.3251056408020904e-67, -3.588778881549252e-68, -7.800551980437032e-68, -6.1581713093038186e-68, -3.2057955965438806e-68, -9.697293041175945e-69, 1.543289763721433e-69, 4.687458556742928e-69, 3.9049483880979624e-69, 2.119134461629086e-69, 6.962896680527191e-70, -4.990995927608514e-71, -2.7915211688805858e-70, -2.4655048668680618e-70, -1.3939932242542608e-70, -4.924344601083624e-71, 3.927467080077828e-74, 1.645151051834821e-71, 1.5497541307447514e-71, 9.12738522750362e-72, 3.4395342160104647e-72, 2.0036221518433227e-73, -9.576080972696221e-73, -9.696289774594392e-73, -5.949722678388557e-73, -2.3773557445591164e-73, -2.5815159823120656e-74, 5.49064253941797e-74, 6.037132757695715e-74, 3.861649169380785e-74, 1.6284201664114956e-74, 2.4807286659373073e-75, -3.089213805414149e-75, -3.7394482624370276e-75, -2.495847697215915e-75, -1.10662502120126e-75, -2.113868432241852e-76, 1.6957758000383484e-76, 2.3034155675194953e-76, 1.6064224235654762e-76, 7.467443963645365e-77, 1.6856322745473272e-77, -8.9991863865603e-78, -1.4103288540622355e-77, -1.0296979156619355e-77, -5.006988869635323e-78, -1.2883079918531505e-78, 4.543678668168596e-79, 8.578181303236732e-79, 6.573027336965598e-79, 3.337715836111659e-79, 9.558195561958412e-80, -2.1141662566815895e-80, -5.179320249526578e-80, -4.178387874942195e-80, -2.212981784556838e-80, -6.936232770225309e-81, 8.37062978236571e-82, 3.101268134330151e-81, 2.6448826446712786e-81, 1.4598632265428433e-81, 4.9474470123399654e-82, -2.0171297916052668e-83, -1.8393258246703207e-82, -1.666895358194387e-82, -9.584554068533997e-83, -3.480086374698044e-83, -8.620554337386052e-85, 1.078753425838644e-83, 1.0457936646429192e-83, 6.2639924737503615e-84, 2.41976985851077e-84, 1.9338340990158314e-85, -6.242663254897406e-85, -6.530250726607995e-85, -4.0758916772113865e-85, -1.6660372835813097e-85, -2.1212445550281623e-86, 3.553529066050428e-86, 4.057380851339728e-86, 2.640825663101548e-86, 1.1373340286341773e-86, 1.9201358446140602e-87, -1.980791993412643e-87, -2.507553882420818e-87, -1.7038804747963386e-87, -7.705826232728537e-88, -1.5855210624222498e-88, 1.07376515097235e-88, 1.5408625136798773e-88, 1.0948173927414702e-88, 5.1858289886466615e-89, 1.2398551494562039e-89, -5.596630177228314e-90, -9.409404031669224e-90, -7.005727804547023e-90, -3.4685955064333816e-90, -9.349806035406329e-91, 2.746903354224976e-91, 5.706407330517513e-91, 4.4644179747537506e-91, 2.3069578551601477e-91, 6.868813994758339e-92, -1.2138795779969215e-92, -3.434061306446763e-92, -2.8330375230661456e-92, -1.5263262897390942e-92, -4.946883853483729e-93, 4.237874744095357e-94, 2.048511947077114e-93, 1.7900930940233344e-93, 1.0048786386264384e-93, 3.5071096818190274e-94, -4.3060744249157035e-96, -1.2096346196217003e-94, -1.1261008749736332e-94, -6.584865467847136e-95, -2.454601117442337e-95, -1.1926497105302533e-96, 7.057562794279636e-96, 7.051483917490095e-96, 4.295681862553622e-96, 1.6995130606122677e-96, 1.704223256475097e-97, -4.058286440295077e-97, -4.394263568065116e-97, -2.7901892763014225e-97, -1.1658611547339225e-97, -1.6912134581197252e-98, 2.2917125095525306e-98, 2.7243850940860876e-98, 1.8046707296049194e-98, 7.93331516254654e-99, 1.4640321662858872e-99, -1.264135623974204e-99, -1.679849218164158e-99, -1.1623984900549929e-99, -5.359700669571324e-100, -1.1785126179286392e-100, 6.754545380554396e-101, 1.0296621849658506e-100, 7.456233050757999e-101, 3.5975966531781505e-101, 9.064356356623966e-102, -3.446031714780245e-102, -6.27040197714801e-102, -4.763114440149107e-102, -2.400573367879994e-102, -6.755774628353267e-103, 1.632505823764485e-103, 3.7910661271982855e-103, 3.0300828140365445e-103, 1.5931007647499802e-103, 4.919622004787324e-104, -6.720717752203688e-105, -2.2735093478656468e-104, -1.9194612442156153e-104, -1.0518489667242896e-104, -3.5187230146787246e-105, 1.8867934935230323e-106, 1.3507962680887472e-105, 1.2106498184386113e-105, 6.911461723173569e-106, 2.4806892083610147e-106, 3.499564060662571e-108, -7.939021964071217e-107, -7.601633824400351e-107, -4.5205484457502814e-107, -1.728136006096324e-107, -1.2245276971436868e-108, 4.6059575691196815e-108, 4.750714340357272e-108, 2.943697244355842e-108, 1.1917729308731339e-108, 1.4238187995466512e-109, -2.630187198456678e-109, -2.954370538273902e-109, -1.9086781895160755e-109, -8.147288751216045e-110, -1.3190768673060703e-110, 1.4721253200341085e-110, 1.827625351172069e-110, 1.2323932656982504e-110, 5.527030632944665e-111, 1.102956901513762e-111, -8.024658050923763e-112, -1.1242243171061093e-111, -7.924402492366014e-112, -3.723783928584415e-112, -8.69349659312024e-113, 4.2163059043247584e-113, 6.873003526379965e-113, 5.074494566054847e-113, 2.4932781828755692e-113, 6.59187025309434e-114, -2.0960524006987115e-114, -4.173467239373314e-114, -3.2360985144614554e-114, -1.6598671924267714e-114, -4.86238292024909e-115, 9.485920605775333e-116, 2.5151354782351553e-115, 2.055095116158086e-115, 1.099183764079932e-115, 3.5128868574873646e-116, -3.519643889725524e-117, -1.5027974940673502e-116, -1.2995296020827136e-116, -7.242757606246731e-117, -2.4967720168809652e-117, 6.027330313111894e-119, 8.890835541183572e-118, 8.181449125009961e-118, 4.74993236124186e-118, 1.7511294687454097e-118, 6.766990903334703e-120, -5.199100208354612e-119, -5.127325047972405e-119, -3.1010550115736987e-119, -1.2145943540309167e-119, -1.11445534976974e-120, 2.997929266567311e-120, 3.197959935133057e-120, 2.015755785938197e-120, 8.344861355595377e-121, 1.1484247836767494e-121, -1.6988751822377609e-121, -1.984523143558719e-121, -1.304734635563432e-121, -5.686078967549086e-122, -1.011771209876774e-122, 9.414526111654497e-123, 1.224867103986753e-122, 8.409982433199977e-123, 3.846117130944748e-123, 8.228265283050459e-124, -5.062707531086727e-124, -7.515921529544322e-124, -5.398509596846767e-124, -2.5844564824598957e-124, -6.371457402896421e-125, 2.6077872940272705e-125, 4.582464573630539e-125, 3.451126601405942e-125, 1.726265172239719e-125, 4.771628787538439e-126, -1.2554824768345657e-126, -2.7742231598869513e-126, -2.1970685195629238e-126, -1.146675011923592e-126, -3.4873939581014118e-127, 5.343034844886365e-128, 1.6662108088251588e-127, 1.3928174542459098e-127, 7.577572861946358e-128, 2.5014793600035293e-128, -1.674402627065458e-129, -9.916906469391172e-129, -8.79161487484383e-129, -4.9831785043130646e-129, -1.7676474580691283e-129, -5.4945043594368865e-132, 5.840355509672869e-130, 5.524654995104655e-130, 3.261909511115221e-130, 1.2338061148670726e-130, 7.594039028417328e-132, -3.3967141837450163e-131, -3.455587478385416e-131, -2.1257210573511932e-131, -8.522865399569494e-132, -9.496977010637329e-133, 1.945571553857245e-132, 2.150868352376052e-132, 1.3793342785871085e-132, 5.834927117573142e-133, 9.034411147966288e-134, -1.0932032542904736e-133, -1.3318289506975367e-133, -8.91259291794898e-134, -3.9634433513241047e-134, -7.659059214436855e-135, 5.990447560363535e-135, 8.200867861179571e-135, 5.735036514885342e-135, 2.6734216596439946e-135, 6.088472743785691e-136, -3.171138379879547e-136, -5.0192688512535614e-136, -3.6751659284665565e-136, -1.7918900495880867e-136, -4.643548307837272e-137, 1.5949875023082195e-137, 3.0516180743323385e-137, 2.3454306111663666e-137, 1.1940871618335481e-137, 3.4398596889161125e-138, -7.371597229613862e-139, -1.8416207482034945e-138, -1.4905767849175834e-138, -7.914556872581214e-139, -2.4933264965264124e-139, 2.8745485965250805e-140, 1.1021238729025582e-139, 9.432740657651363e-140, 5.219526935923913e-140, 1.7767703020863988e-140, -6.468720635308747e-142, -6.532444503865085e-141, -5.943223720700097e-141, -3.42584355873268e-141, -1.248841708652143e-141, -3.5471401511139855e-143, 3.828378114884239e-142, 3.727667506344888e-142, 2.238352590698876e-142, 8.677832253112392e-143, 7.203634072372229e-144, -2.2134456174693487e-143, -2.3269776769460355e-143, -1.456080387561231e-143, -5.971465290143648e-144, -7.763501751701188e-145, 1.258538465463676e-144, 1.4453448361413413e-144, 9.431713578967766e-145, 4.074488719391991e-145, 6.975602781443014e-146, -7.004967691810509e-146, -8.929547802976853e-146, -6.083869175282321e-146, -2.7594109319329634e-146, -5.736411843060109e-147, 3.7896954879010466e-147, 5.485096451855891e-147, 3.908166699459078e-147]
  out "Noise check J8":dbl[](graph)=[0.0, 0.0, 0.0, 0.0, 0.0, 0.0, 0.0, 0.0, 0.0, 0.0, 0.0, 0.0, 0.0, 0.0, 0.0, 0.0, 0.0, 0.0, 0.0, 0.0, 0.0, 0.0, 0.0, 0.0, 0.0, 0.0, 0.0, 0.0, 0.0, 0.0, 0.0, 0.0, 0.0, 0.0, 0.0, 0.0, 0.0, 0.0, 0.0, 0.0, 0.0, 0.0, 0.0, 0.0, 0.0, 0.0, 0.0, 0.0, 0.0, 0.0, 0.0, 0.0, 0.0, 0.0, 0.0, 0.0, 0.0, 0.0, 0.0, 0.0, 0.0, 0.0, 0.0, 0.0, 0.0, 0.0, 0.0, 0.0, 0.0, 0.0, 0.0, 0.0, 0.0, 0.0, 0.0, 0.0, 0.0, 0.0, 0.0, 0.0, 0.0, 0.0, 0.0, 0.0, 0.0, 0.0, 0.0, 0.0, 0.0, 0.0, 0.0, 0.0, 0.0, 0.0, 0.0, 0.0, 0.0, 0.0, 0.0, 0.0, 0.0, 0.0, 0.0, 0.0, 0.0, 0.0, 0.0, 0.0, 0.0, 0.0, 0.0, 0.0, 0.0, 0.0, 0.0, 0.0, 0.0, 0.0, 0.0, 0.0, 0.0, 0.0, 0.0, 0.0, 0.0, 0.0, 0.0, 0.0, 0.0, 0.0, 0.0, 0.0, 0.0, 0.0, 0.0, 0.0, 0.0, 0.0, 0.0, 0.0, 0.0, 0.0, 0.0, 0.0, 0.0, 0.0, 0.0, 0.0, 0.0, 0.0, 0.0, 0.0, 0.0, 0.0, 0.0, 0.0, 0.0, 0.0, 0.0, 0.0, 0.0, 0.0, 0.0, 0.0, 0.0, 0.0, 0.0, 0.0, 0.0, 0.0, 0.0, 0.0, 0.0, 0.0, 0.0, 0.0, 0.0, 0.0, 0.0, 0.0, 0.0, 0.0, 0.0, 0.0, 0.0, 0.0, 0.0, 0.0, 0.019514023343214733, 0.08249592275615225, 0.17521572873906943, 0.2877229529743026, 0.4292775162061891, 0.580089642599734, 0.7266039469351937, 0.9105187417916951, 1.1561228694312586, 1.4161073383424392, 1.6712653415602594, 1.9429161747507073, 2.1762441029636683, 2.3003504374189507, 2.338588131429958, 2.329341968477711, 2.25398808993314, 2.107931197896546, 1.9635101814896299, 1.9063659590150102, 1.9503238507958631, 2.078058753847821, 2.28023393793774, 2.478628536044209, 2.5440501184382733, 2.447849145968754, 2.282169773547936, 2.1289520790388763, 2.0157325897382687, 1.9747777958778192, 2.0167473869964656, 2.0463574231853516, 1.916033217173922, 1.6017833261308014, 1.2335278380792691, 0.910359687462185, 0.6126309141606225, 0.33927728264581225, 0.17909516336600512, 0.17010659494479582, 0.2226103777184982, 0.22742785008742636, 0.16075864104743492, 0.07575541692949156, 0.01783667834746522, -0.008435224025382628, -0.013898364928056059, -0.010291762775584083, -0.005070378689286361, -0.0013498112806428306, 0.0004175119499425963, 0.0008435711349220477, 0.0006561558432412835, 0.0003374392833874356, 9.94221929488852e-05, -1.8743618683019793e-05, -5.081238414927928e-05, -4.165850230594167e-05, -2.233855124971594e-05, -7.174820658762593e-06, 6.816979610941673e-07, 3.034317887601836e-06, 2.633549685767141e-06, 1.4714951593295828e-06, 5.094890456044555e-07, -1.0147507660297524e-08, -1.7939684383980361e-07, -1.6575446385001977e-07, -9.647585925378466e-08, -3.570682444886013e-08, -1.5060971853072481e-09, 1.048231277247774e-08, 1.0384851653685573e-08, 6.296827777090617e-09, 2.475088943630927e-09, 2.345936424114962e-10, -6.038526407137477e-10, -6.475156102519583e-10, -4.091993583398243e-10, -1.6995831810171214e-10, -2.383845288509984e-11, 3.417766378317056e-11, 4.0169161396624976e-11, 2.647929396311701e-11, 1.15751972975944e-11, 2.08676934922926e-12, -1.89097408904847e-12, -2.4784172516287225e-12, -1.7063494972990366e-12, -7.826226502762988e-13, -1.6908054506106593e-13, 1.0146355011956984e-13, 1.5202093413076725e-13, 1.0950552783504866e-13, 5.256915703584442e-14, 1.3060833950058552e-14, -5.209180006564298e-15, -9.264873326103514e-15, -6.998613005441442e-15, -3.510064511362837e-15, -9.764495560353943e-16, 2.494160337086511e-16, 5.606348770411843e-16, 4.45432953197793e-16, 2.330799233464178e-16, 7.127220807632587e-17, -1.0497225594261098e-17, -3.365428189390463e-17, -2.8230486059437765e-17, -1.5397863540459433e-17, -5.1070829471793616e-18, 3.176172014428728e-19, 2.001813351675452e-18, 1.7814553270383526e-18, 1.0123010722811393e-18, 3.605881614037581e-19, 2.5320880985356465e-21, -1.1780877824787093e-19, -1.1191521067600754e-19, -6.624507976661101e-20, -2.515138993895e-20, -1.6312645872611888e-21, 6.845825644234186e-21, 6.998061176898739e-21, 4.3158934697131486e-21, 1.7363763267842923e-21, 1.9844014391023203e-22, -3.9170094703668483e-22, -4.354459090991873e-22, -2.7997535787307327e-22, -1.1881466245651159e-22, -1.8694418745495592e-23, 2.197962046512941e-23, 2.695405782023135e-23, 1.8085989265196698e-23, 8.066948265106462e-24, 1.57692867391821e-24, -1.2022401433353857e-24, -1.659125768595587e-24, -1.1634920613085807e-24, -5.439089123454862e-25, -1.2497155325352989e-25, 6.347866043384645e-26, 1.0150543942239129e-25, 7.454069257924207e-26, 3.644249245536799e-26, 9.511413858293039e-27, -3.180050501295051e-27, -6.168651651406225e-27, -4.755843717550897e-27, -2.427635240122828e-27, -7.035152148674132e-28, 1.459312412400644e-28, 3.72090365312897e-28, 3.0216641362255066e-28, 1.6085510505480058e-28, 5.093350955611504e-29, -5.5977950225885286e-30, -2.225548827892454e-29, -1.9116743899997508e-29, -1.0604942901551555e-29, -3.626188086378487e-30, 1.1617805286905463e-31, 1.3182630808045061e-30, 1.204144334143296e-30, 6.958571386652768e-31, 2.5467895726861447e-31, 8.161244058449303e-33, -7.719849106734093e-32, -7.550385006093093e-32, -4.5452882155921776e-32, -1.7685438242256757e-32, -1.523030360500267e-33, 4.459219286268611e-33, 4.711869048324583e-33, 2.9559863127548837e-33, 1.2163076063499341e-33, 1.6141703769346005e-34, -2.5325042618052453e-34, -2.9257247081866263e-34, -1.9142316207899795e-34, -8.295133103675373e-35, -1.4399544219718923e-35, 1.4074423193906177e-35, 1.806934151550668e-35, 1.2344464158285114e-35, 5.6153585834146886e-36, 1.1793894580737767e-36, -7.598471498530369e-37, -1.1095205824597296e-36, -7.927836536800844e-37, -3.776034025548034e-37, -9.174668416745864e-38, 3.9368197483347213e-38, 6.769892059390753e-38, 5.070442194683307e-38, 2.5238280595030366e-38, 6.89340515670207e-39, -1.913595489316326e-39, -4.1019568481587746e-39, -3.229496841518112e-39, -1.6774798725577334e-39, -5.050442437466536e-40, 8.299967811592404e-41, 2.4660092822497864e-40, 2.0483102542106454e-40, 1.1091623335517886e-40, 3.629581919180045e-41, -2.7520512794023853e-42, -1.4693265226384872e-41, -1.2935592879331514e-41, -7.298038849396681e-42, -2.5687927199178417e-42, 1.0798614176838713e-44, 8.664452710550936e-43, 8.132928975278173e-43, 4.779648068920027e-43, 1.795319089865324e-43, 9.942704747656584e-45, -5.046989772830594e-44, -5.089771082185439e-44, -3.116352271590489e-44, -1.2415347376818345e-44, -1.3174608559448551e-45, 2.896335118690861e-45, 3.169844556001687e-45, 2.02311306824445e-45, 8.507944408831343e-46, 1.277656686442252e-46, -1.6313951935949141e-46, -1.9639797010622222e-46, -1.307859421780129e-46, -5.784017876185206e-47, -1.09369294440593e-47, 8.968623620279824e-48, 1.210134258776604e-47, 8.419714000267961e-48, 3.904401624399035e-48, 8.745338200284505e-49, -4.769488154408877e-49, -7.411829289123403e-49, -5.3981102836453414e-49, -2.6187774198368084e-49, -6.696369347646424e-50, 2.415860499388664e-50, 4.509818237906732e-50, 3.446610577460599e-50, 1.7462228692733178e-50, 4.974845172813906e-51, -1.1304138881778935e-51, -2.7240461587753553e-51, -2.191450718787662e-51, -1.1581041655960669e-51, -3.61387505488602e-52, 4.531531417591415e-53, 1.6318618975671771e-52, 1.3874831043865497e-52, 7.641776500022628e-53, 2.5797922966821662e-53, -1.1500733062517325e-54, -9.68360716722353e-54, -8.746434623636637e-54, -5.018348589029852e-54, -1.8158662156690544e-54, -3.9232223426238247e-56, 5.683002435887264e-55, 5.488760157974862e-55, 3.280518558718337e-55, 1.263315838912452e-55, 9.755940906104331e-57, -3.2912538668332935e-56, -3.428221933995834e-56, -2.1350740136434545e-56, -8.70226439844676e-57, -1.0876601782817839e-57, 1.8752989492294287e-57, 2.1306021977634424e-57, 1.3836513663228454e-57, 5.943182859787397e-58, 9.911153149069492e-59, -1.0466284731177401e-58, -1.3171425592682841e-58, -8.929377562247632e-59, -4.0282227038261215e-59, -8.21385599257535e-60, 5.683311316700688e-60, 8.096229293036184e-60, 5.738761074629174e-60, 2.711812730960853e-60, 6.438012036175147e-61, -2.9695598123494333e-61, -4.945731852660163e-61, -3.673027437145264e-61, -1.814386193499494e-61, -4.86277229104564e-62, 1.463288295179092e-62, 3.0005255321512638e-62, 2.3411598361503453e-62, 1.2070914839275723e-62, 3.576701530135096e-63, -6.514917381068056e-64, -1.806466144581475e-63, -1.4859887017210366e-63, -7.988482021442263e-64, -2.578317405928066e-64, 2.319663781033632e-65, 1.0781391339282496e-64, 9.39157197516554e-65, 5.2606618597606215e-65, 1.8292755743663787e-65, -2.8896402195696983e-67, -6.370023140480876e-66, -5.909394071280015e-66, -3.448089113847277e-66, -1.2810915689558914e-66, -5.846167635707302e-68, 3.7191232592980426e-67, 3.701295290147923e-67, 2.2499069120172192e-67, 8.874674826518393e-68, 8.674339608182023e-69, -2.1404003609380556e-68, -2.3071334665039774e-68, -1.461719505377166e-68, -6.09077877091794e-69, -8.700429442402992e-70, 1.2099752359115472e-69, 1.4307899072545627e-69, 9.456365825267808e-70, 4.1462475097215744e-70, 7.56997699046677e-71, -6.6837822812250005e-71, -8.82485603019384e-71, -6.092226628851743e-71, -2.8021876723171554e-71, -6.111856640531614e-72, 3.578311872843938e-72, 5.410950334161581e-72, 3.908722274317711e-72, 1.8815285898727497e-72, 4.7101474175460734e-73, -1.830992393795656e-73, -3.2963253231205535e-73, -2.4974745207020884e-73, -1.2558664515319068e-73, -3.5155073862316743e-74, 8.717693556186078e-75, 1.9937478260619503e-74, 1.589133691839586e-74, 8.336670042617291e-75, 2.5627755867339513e-75, -3.6268201948721746e-76, -1.1961984161031075e-75, -1.0068926757324135e-75, -5.5057471321557316e-76, -1.8345592577528926e-76, 1.0560998852440493e-77, 7.110898046464844e-77, 6.352185676893933e-77, 3.6185987411620635e-77, 1.2942523853937532e-77, 1.4033270651028862e-79, -4.181867673451595e-78, -3.9894802220666727e-78, -2.3673621334267444e-78, -9.021436834048458e-79, -6.142851037798668e-80, 2.4279920613966517e-79, 2.49389456963419e-79, 1.541935661871305e-79, 6.224526936720257e-80, 7.287547359399441e-81, -1.3877657581001573e-80, -1.5513163496481292e-80, -1.0000064947689516e-80, -4.25709715026244e-81, -6.802747015974906e-82, 7.776632439951589e-82, 9.599461716105041e-82, 6.458248486947503e-82, 2.889074494242771e-82, 5.7109605932704264e-83, -4.245903030688349e-83, -5.906729298103802e-83, -4.153616778200488e-83, -1.9471576877197778e-83, -4.512589473014001e-84, 2.236015469626954e-84, 3.612332092886322e-84, 2.6604008684946296e-84, 1.3041392954207359e-84, 3.427540297069213e-85, -1.1156150022720623e-85, -2.1943253434230985e-85, -1.6969581065279417e-85, -8.684656648794885e-86, -2.5314457897597907e-86, 5.082155707379183e-87, 1.3229654984177616e-86, 1.0778986433634132e-86, 5.752640873994785e-87, 1.83064635109878e-87, -1.9159702624311993e-88, -7.908548590485092e-88, -6.817594362756693e-88, -3.7915067435508826e-88, -1.3021353847869056e-88, 3.6170567042594108e-90, 4.681470659092097e-89, 4.293164308484522e-89, 2.487143907339247e-89, 9.13846994060342e-90, 3.2535239509598085e-91, -2.7394114670709364e-90, -2.69119269813339e-90, -1.6241436527494756e-90, -6.341930879291941e-91, -5.65417598253341e-92, 1.5808961358611156e-91, 1.678955703443119e-91, 1.0559692390015737e-91, 4.3592544501550785e-92, 5.900470468244734e-93, -8.96783126013451e-93, -1.0421775884851994e-92, -6.836467446868863e-93, -2.971558026438741e-93, -5.227892926225754e-94, 4.976288702193919e-94, 6.434320957359681e-94, 4.407573074308357e-94, 2.0107260934383415e-94, 4.2653971626919655e-95, -2.680965300536676e-95, -3.9494373797444063e-95, -2.8299101706063056e-95, -1.3515857691311949e-95, -3.3098389340843546e-96, 1.3847398238689153e-96, 2.4088248708771516e-96, 1.8094819265610855e-96, 9.030542973154048e-97, 2.4824711436147173e-97, -6.696847513848296e-98, -1.458875219820159e-97, -1.1522124973248558e-97, -6.000246203616696e-98, -1.8163780480720846e-98, 2.8758442121869184e-99, 8.765965419004886e-99, 7.306016717837865e-99, 3.966190146525619e-99, 1.3040210248320863e-99, -9.262056955040729e-101, -5.21997185352633e-100, -4.612701428473814e-100, -2.6089059950414993e-100, -9.221330179381699e-101, 2.3998482703849025e-104, 3.0760393251083094e-101, 2.89931773855064e-101, 1.7081565366220336e-101, 6.440261809812088e-102, 3.780819423730534e-103, -1.7902948628758058e-102, -1.813933497941581e-102, -1.1134279483959655e-102, -4.451054375840228e-103, -4.8506781546235494e-104, 1.0263584697483747e-103, 1.129349317003883e-103, 7.226412572596635e-104, 3.0486293883001276e-104, 4.6547116085660915e-105, -5.773593770487325e-105, -6.994966945426022e-105, -4.67038682488621e-105, -2.0716272777131214e-105, -3.96353319920563e-106, 3.1685693222219886e-106, 4.3085335389389837e-106, 3.0059346023972412e-106, 1.3978444752315084e-106, 3.1592220917471986e-107, -1.6809384316399712e-107, -2.637877982275337e-107, -1.9267024017327793e-107, -9.37219784033095e-108, -2.4138515242506406e-108, 8.482649046768349e-109, 1.6043689965362803e-108, 1.2298586277427348e-108, 6.247321685914655e-109, 1.7905026120095856e-109, -3.943385103926138e-110, -9.686201170453539e-110, -7.817776340777646e-110, -4.141936495666987e-110, -1.2991297308476788e-110, 1.5581424212439851e-111, 5.799463198980326e-111, 4.948405533239757e-111, 2.7322470784930444e-111, 9.265187383595001e-112, -3.721878244380564e-113, -3.439297840578624e-112, -3.1185384926451727e-112, -1.7937536738613592e-112, -6.516543512058082e-113, -1.6467723016009456e-114, 2.0169219891483998e-113, 1.956464697588156e-113, 1.1722652767060967e-113, 4.5306740281515506e-114, 3.6400951584865278e-115, -1.1670332132864976e-114, -1.2216259705959625e-114, -7.627489394138378e-115, -3.119179396711746e-115, -3.982940728235264e-116, 6.642112125040166e-116, 7.589890276101473e-116, 4.9417798019108615e-116, 2.1291912533820195e-116, 3.601608309757262e-117, -3.701675299263825e-117, -4.690509044399344e-117, -3.1883625702608684e-117, -1.4425140442839912e-117, -2.972277601397658e-118, 2.0060899509237447e-118, 2.88211894442371e-118, 2.04859114940971e-118, 9.707239433605624e-119, 2.3234359421062925e-119, -1.0451900641139902e-119, -1.7598932899871703e-119, -1.310846617981511e-119, -6.49246946897847e-120, -1.7516701909433598e-120, 5.1266599576831154e-121, 1.0672361997698223e-120, 8.353112733905654e-121, 4.317936211647777e-121, 1.2866183900142392e-121, -2.2627661937807715e-122, -6.422084393196871e-122, -5.300543833782142e-122, -2.8567058540595657e-122, -9.264801637537202e-123, 7.874140945308415e-124, 3.830648340305231e-123, 3.3490985255174815e-123, 1.880677590905294e-123, 6.567536618337897e-124, -7.699239832739094e-126, -2.2617680020554507e-124, -2.10675118952308e-124, -1.2323414024943094e-124, -4.5961222007986203e-125, -2.2546089214795788e-126, 1.3194741659592869e-125, 1.3191658045163532e-125, 8.038967258574651e-126, 3.1819916679785086e-126, 3.2035476195071124e-127, -7.586305232451694e-127, -8.220286371859143e-127, -5.221391904965381e-127, -2.182680040358373e-127, -3.173865086087825e-128, 4.283251434602674e-128, 5.096243208608686e-128, 3.377033696976561e-128, 1.4851501670339075e-128, 2.7453510659449232e-129, -2.362158749489864e-129, -3.142181648652864e-129, -2.1750910188131988e-129, -1.0033015959167371e-129]
  out "Noise check J4 2":dbl[](graph)=[0.11715728752538133, 0.3740608468982666, 0.48935145067047375, 0.5124139545254041, 0.7202787581809311, 1.0452515753220093, 1.2725875104120554, 1.3395451839359782, 1.3366579462013999, 1.2823272859707244, 1.2320662608483122, 1.232079253881954, 1.297660715341265, 1.5059337885607809, 1.6218563941944275, 1.4469365567065449, 1.3898262932330816, 1.609077193422325, 1.678615962286397, 1.4465426411585365, 1.1557466895989457, 1.1151491276228955, 1.4666985817923337, 1.9288323939305854, 2.081380355051217, 1.9344758459116282, 1.8818071281850481, 2.076380900492726, 2.2578568369337626, 2.4031484957125118, 2.479638806461897, 2.415456044459552, 2.2903947567051097, 2.027907273864818, 1.9002236560092767, 2.062600360122229, 2.2582517908540636, 2.3885881607088524, 2.5341212907216866, 2.6474119995168244, 2.6080813878206914, 2.552762776491808, 2.6406384882810467, 2.8102697920575026, 2.9213816004759874, 3.008647479329108, 3.1710425569859897, 3.3243508001062954, 3.3659439688479775, 3.422397387755387, 3.4519946846551703, 3.129135829487624, 2.6000874555843696, 2.413940736792694, 2.697919496742492, 3.086284789267005, 3.3187270826707187, 3.340078929973166, 3.0874667343208504, 2.8812368189869293, 2.956504493964696, 3.086447736290119, 3.1838701750544263, 3.330037590003737, 3.5622917989670193, 3.7813562319422274, 3.939763412267218, 4.152773158583681, 4.310561387208063, 4.1247184101060865, 3.7602243926587446, 3.5468655474972843, 3.4672069049933296, 3.472986738948049, 3.583093757844309, 3.7045032540706746, 3.8408455289774217, 4.036314606665514, 4.097052337140383, 3.9231872353736117, 3.7390197352540238, 3.681918628660658, 3.6601830339052746, 3.47322518226167, 3.118705789007265, 2.8663071980995913, 2.7660428701816286, 2.9411446574901667, 3.334915794276792, 3.3939587302787677, 3.123105752711805, 2.9652194253803006, 3.0042781672234447, 3.171836736313404, 3.3167928896315892, 3.260922503136668, 3.1111131433509356, 3.0470736303589865, 3.134264124691393, 3.403787439412938, 3.6483591739263375, 3.7012345459897604, 3.7476668716939603, 3.9007389589875863, 3.9905268358253276, 3.6531575516708243, 3.0024971218314094, 2.628425408449802, 2.600028205051599, 2.6198407777090753, 2.5894073410509235, 2.593162660092505, 2.763057404425491, 2.9903256835425145, 2.9819918665202225, 2.7714581806225462, 2.536690627832922, 2.3269489079293058, 2.1391166178806076, 2.031940543156169, 2.1301882363272044, 2.3659365882365155, 2.457821961959852, 2.163213213018353, 1.7376676753539695, 1.58110902055965, 1.5948788324240004, 1.5721793881713308, 1.634056175246943, 1.9830907625031058, 2.5063264919644097, 2.7856619332227743, 2.6891109644731874, 2.4561544879408697, 2.3272833155836534, 2.615380215918678, 3.2521401765535103, 3.6783460662955387, 3.7214769031015145, 3.6200724160991786, 3.461274866825482, 3.2770188462001393, 3.165996227706985, 3.2496621675324677, 3.4729448918017107, 3.5286488216441727, 3.4969763083011025, 3.5657044872628534, 3.4457973943715174, 3.163391900649769, 3.1128424100283087, 3.3155287744974524, 3.552762463612855, 3.7088664091890107, 3.7086229730765696, 3.6173063816081994, 3.658213813715342, 3.8443778619220312, 4.006259199086435, 4.0968277046928705, 4.128256064939727, 4.127697505273751, 4.214325843025934, 4.4231064044904045, 4.45438699084868, 3.95541904719735, 3.3378771942308965, 3.2636845548649234, 3.526502742793165, 3.6232850551647124, 3.519532051459479, 3.45779376174084, 3.5903803952512123, 3.8531209895493146, 4.212849369641261, 4.513239877275157, 4.471516050677759, 4.312522065913468, 4.410843616770427, 4.63464491717242, 4.646900132429299, 4.378828773543272, 4.004846313318664, 3.683030744291786, 3.5140440434600166, 3.5205723541136837, 3.6318717411703854, 3.754155920646328, 3.851872969600686, 4.0008711666507395, 4.1478280935326275, 4.148846381592598, 3.9250848592004415, 3.5673344339709017, 3.382736130915638, 3.464628825590554, 3.7205280537800522, 4.012599453309597, 4.212430374137527, 4.1179766013234, 3.640131882665263, 3.1722846159112676, 2.890475555622189, 2.6342859050931726, 2.5062105542319255, 2.6075400077254307, 2.843397189215909, 3.1686724900623044, 3.5138832117321677, 3.6723472573287625, 3.540705527731992, 3.256376986054855, 2.9736113989513724, 2.7822674127534315, 2.647306231745915, 2.486213865824263, 2.5160050891522685, 2.7832890177547736, 2.8496203832467155, 2.81330044421172, 2.8936307242487818, 2.786211339049903, 2.6581586114308564, 2.77826105693475, 2.9634682928929665, 3.2249695958386617, 3.595278681903802, 3.8767685500316738, 3.9503816297381884, 3.7697450341210605, 3.4577442377717444, 3.145694406181593, 2.9554912689840074, 2.9778137149647184, 3.1794178521234704, 3.547550278712043, 3.866479909121504, 3.878486015442823, 3.6663383167082224, 3.559952585687788, 3.6279981291024233, 3.688561563838123, 3.752268791772671, 3.8604864817614, 3.9803317848721793, 4.1939339590195335, 4.365134693030768, 4.269844529684406, 4.142463405358109, 4.249392863274142, 4.412193512371845, 4.334778137802275, 4.100129159436453, 3.9925730715357224, 4.01820008197657, 4.029397951960254, 3.943545102569681, 3.6440812761275723, 3.351309260219587, 3.370364577855667, 3.5054469901700713, 3.567873493550758, 3.610991616482299, 3.6894135819406633, 3.8173195634460724, 3.999637789773048, 4.099604412949512, 3.937818961152086, 3.742200859381764, 3.7581454376747834, 3.8871997006460015, 4.003558367198969, 4.099533604315813, 4.385548278503996, 4.740371041173527, 4.803826993960021, 4.579406761771866, 4.278327602432292, 4.235247016832022, 4.373094829341549, 4.351446364543641, 4.285086725359295, 4.288317056235496, 4.352534950296121, 4.44129270637045, 4.405937283683173, 4.343017952813209, 4.383350145318506, 4.325191523843934, 4.139757697977947, 4.101472505019914, 4.20529301257928, 4.159727940093391, 3.8673735814570334, 3.509296533346232, 3.2789128149769193, 3.161537763714405, 3.000749682098558, 2.878519134766226, 2.8949799551393136, 2.9512428811963636, 2.9499855999955416, 2.8324148422880944, 2.6341191969854307, 2.466828307669313, 2.433782136844685, 2.360758465035781, 2.1174274386978507, 1.9221170781990922, 1.7995608319312884, 1.7686433629347937, 2.004897643468315, 2.452734498729815, 2.835260137354656, 2.880656992338984, 2.688554831237719, 2.560648642905691, 2.4064605128345606, 2.2256210874592885, 2.3505977678425616, 2.655627115372408, 2.8527371122414253, 2.975950179474258, 3.036176348306544, 3.17880749722969, 3.5665730486607954, 3.8065133419061254, 3.620345924487635, 3.3355561804677127, 3.20721449901231, 3.132327179528711, 3.0556877616359515, 3.0279200799204995, 3.046813145753882, 3.1910388804753302, 3.3304816258821845, 3.3748218329525175, 3.409197695123555, 3.3584857487106703, 3.308978553686482, 3.3573115630821952, 3.4193827596887396, 3.295820217945015, 2.9828980062312485, 2.875506239036952, 3.1128782888900446, 3.411524488616971, 3.653019238511069, 3.771390831669732, 3.714626424357457, 3.6899929812403167, 3.783320890386088, 3.928337971135291, 3.9363210100630663, 3.651430782082533, 3.2239629696076784, 3.0135369332857427, 3.289580282470677, 3.776188176758647, 4.006268547357298, 4.060987769618934, 4.172567592362272, 4.181421458998683, 3.986602866274385, 3.79997484670682, 3.796353973585663, 3.9137281652871603, 4.035359679472552, 4.052331596457997, 3.9789734987141463, 3.9920214808702044, 4.067828364844418, 4.213055311434371, 4.422338701373815, 4.424797382058289, 4.240197030932777, 4.202018092697205, 4.334950275137475, 4.375375178466772, 4.222730805943901, 3.9774733779622493, 3.75807148567848, 3.808705805175082, 4.17365594584997, 4.48132991711847, 4.591179028435549, 4.52384602231574, 4.316353304678457, 4.211513380857337, 4.123254948209748, 3.830913058842902, 3.5358944233949448, 3.4918789850279683, 3.734219415497558, 3.967608869980387, 3.872555839336078, 3.4903541373240365, 3.03477486568797, 2.664309425512988, 2.505943445309487, 2.577754120290767, 2.6396678902503723, 2.635051431531166, 2.7272183567161195, 2.952336488801323, 3.2021993418168044, 3.3334435995522123, 3.334841825553929, 3.2924119997587202, 3.232416486444775, 3.0630750544839356, 2.7769703163480575, 2.592964648262377, 2.622244866965743, 2.6721333154188756, 2.582488127970704, 2.471577244598757, 2.631205765145985, 2.935832559594978, 2.935513373809811, 2.8531963923368417, 3.117402348472467, 3.374410891993727, 3.2552852143183086, 3.0377767192266854, 2.891942517246099, 2.836714652037887, 2.9992295460267933, 3.2782535261056207, 3.594542406244116, 3.916891716356328, 4.125139041058814, 4.155448087873499, 3.890056488594309, 3.346609762109395, 2.9227071411876406, 2.860406542961092, 3.0210747076479674, 3.203084079378447, 3.2234970328651738, 3.055152364581866, 2.821289420336848, 2.774073498964793, 2.8172753234307146, 2.766350854375779, 2.8503848057644365, 2.9075351687767146, 2.777196013924327, 2.7914706759537466, 3.0729268090883886, 3.343291082833762, 3.406743180658967, 3.2495245727949644, 3.0508574266394266, 3.2381409882948162, 3.676198151490693, 3.8608017278021345, 3.840013057789408, 3.876036073827179, 3.868112919254649, 3.7217148306540597, 3.605856655162829, 3.4868452388726663, 3.423022698667008, 3.646598385145646, 4.034871460604682, 4.355702919805467, 4.5287613618775895, 4.575215498757915, 4.492984980613729, 4.224236661031898, 4.008031595428675, 4.118325745693038, 4.431063925109908, 4.728204020732383, 4.786947042170808, 4.6847051516092915, 4.783517926076508, 4.940049455336525, 4.898481488225954, 4.787587441986354, 4.784759487214933, 4.867873484436023, 4.644520437981334, 4.191448140115397, 3.9461326769135256, 3.6901352081674794, 3.4231561208472767, 3.4032249223972073, 3.356269349870267, 3.191722549536731, 3.0620013032216393, 3.0433634092238973, 3.156899815329176, 3.016314807248221, 2.6213730540598705, 2.4520897843164486, 2.502240096426813, 2.4887927331783883, 2.30318795011837, 2.2107853952549013, 2.3026929796097293, 2.3225140598127685, 2.251987048227818, 2.13983408812029, 2.0966566963274977, 2.2885951268647995, 2.552290629589841, 2.483084867299442, 2.0565715437482375, 1.8044399081982432, 2.0506077856655973, 2.5717662179749654, 2.9127213898407156, 2.865195385337823, 2.628630856276723, 2.440963895448842, 2.342884630994453, 2.254391623521738, 2.164600274936008, 2.236362243610271, 2.6463699594476893, 3.1359286796520265, 3.4022411850708556, 3.5096629975855507, 3.3952500237287646, 3.0758372353759897, 2.871408272235008, 2.843720370638062, 2.7686016668583067, 2.755823910744054, 2.8762106749065883, 2.9061036910398794, 2.9136843901305554, 2.988972061413916, 3.076953273510197, 3.0859913288672245, 2.8308708434266285, 2.4115923266533503, 2.257542628612427, 2.447324831913182, 2.745944859519945, 3.0423306454617576, 3.1734102985729398, 3.1103301530689627, 3.1047954767775914, 3.325629302265265, 3.682124931126049, 3.9153316362565787, 3.8601594334237683, 3.7108807987845873, 3.5787671793155638, 3.425863950893511, 3.4819529945069614, 3.702959282292147, 3.7949985878535415, 3.671421812609753, 3.4558909920034147, 3.38174680965479, 3.549659435018868, 3.849840991382825, 3.998779143367324, 3.8731660369125587, 3.548881097043789, 3.226434715408849, 3.17697094074099, 3.296396817727691, 3.318086359007308, 3.3182530435588267, 3.4088114211056997, 3.5331875459058484, 3.678842998838103, 3.764946461257866, 3.6901795862630564, 3.366436078610211, 2.9494465619936054, 2.634930256152137, 2.4676348375248995, 2.756454728124067, 3.3578888761380075, 3.6529172006472965, 3.4767537335411562, 3.007297195951196, 2.5257794104458022, 2.3259166740565487, 2.3175164222027904, 2.298112642582997, 2.3314342041367486, 2.3107393564265, 2.153200484887369, 2.0896745533199788, 2.0530053659616847, 1.9029251329823331, 1.8810453750510217, 1.9983116514162438, 2.0380597513395546, 2.0754982897196763, 2.22446671038613, 2.2840942204508177, 2.0661039680877007, 1.7723631994382978, 1.6657162372665657, 1.633792784742251, 1.580665408691699, 1.6290855546811824, 1.7607873825214464, 1.9664480808767877, 2.2336035250295767, 2.4462158490475945, 2.577143070353526, 2.639474771011086, 2.5960206111035524, 2.5538006172834193, 2.5772954818123432, 2.525652018150299, 2.3812625065174347, 2.2623452573276994, 2.2471743732714136, 2.409193711790544, 2.762266116285253, 3.050902632696721, 3.039368124607681, 2.8639393628975056, 2.7219145908208495, 2.558620639837702, 2.3934285733446576, 2.545956106090098, 2.959612825680251, 3.0937443569364618, 2.7796628780621115, 2.350965543923136, 2.2272155787743024, 2.4779935718731574, 2.8044948560484184, 2.7456004429710523, 2.259057955736487, 1.9468931655028632, 2.019787461054642, 2.192567792058492, 2.3018792299378603, 2.366871812838477, 2.4795782273171945, 2.564174659631819, 2.5575485996084844, 2.6402599670622573, 2.7985545371639877, 2.8128314530397227, 2.5977910704246248, 2.341474544962357, 2.3569961733698523, 2.5547000197310887, 2.7359231175001817, 2.850643717793762, 2.7714752429307428, 2.7074098253926744, 2.985817295507075, 3.5332614116863827, 4.00540972061191, 4.1118643264743024, 3.9376906342321982, 3.70870391187847, 3.5801603789365144, 3.613402139643432, 3.6778275092162223, 3.8055926016046646, 4.090074601297982, 4.276646009471579, 4.260088813829417, 4.31897157279649, 4.43858447932069, 4.375519306058752, 4.1687957414254555, 4.043732156470664, 4.072833791030641, 4.073617185813728, 4.0353659107636775, 3.920936272849831, 3.669591683915871, 3.480528052847939, 3.3665324670998484, 3.18539410639914, 3.072139965323421, 3.2502938584445045, 3.407194803561768, 3.2321339052786247, 2.965969056041802, 2.9295897790915575, 3.0718806499129596, 3.0424242638199717, 2.771960080529735, 2.6439400859893, 2.896526516916376, 3.138288190113719, 2.959845263841691, 2.5450476111526563, 2.3208477894260264, 2.423471985898821, 2.7121175676527223, 2.930520951864521, 2.9328242630619634, 2.8231422884387647, 2.7482546825476346, 2.792315487169028, 2.8392927328549398, 2.80055461890597, 2.767899107513304, 2.7890763299395935, 2.946847972002077, 3.1471160722644296, 3.146656598465134, 2.9623100814666277, 2.8081858909769375, 2.7243250496562434, 2.599003947449827, 2.4111726200243355, 2.227041710501784, 2.262498476051084, 2.3573044050370697, 2.2981858681179324, 2.4158716538262213, 2.7613214160939283, 2.901339370729471, 2.7327006050059315, 2.6539541951945225, 2.8116602212281188, 2.8401490823483155, 2.5117836367450472, 2.1243596875906228, 1.936889784993296, 2.0357293915915626, 2.357379057885556, 2.5202925557250317, 2.420225709645792, 2.4375501071141477, 2.5946335012786172, 2.619801058897777, 2.610694342975067, 2.583956155697185, 2.473914757306284, 2.4669474266916693, 2.643505639929545, 2.8025256559802125, 2.776441139633968, 2.5914475695289454, 2.503833656131722, 2.629341599187499, 2.8354549042526163, 3.1148648056589425, 3.231485693640419, 2.8480128884195213, 2.183993734197156, 1.7345902766885133, 1.7079642829933193, 1.9400563881308628, 2.1384609326847386, 2.287206925310381, 2.4687053241039063, 2.570715443389662, 2.4794716451014684, 2.2520486137602216, 2.048520508389529, 2.0300711204815394, 2.1781506454782806, 2.2360431908436773, 2.06552903310072, 1.7780750481095127, 1.4760309189579577, 1.1406323686274344]
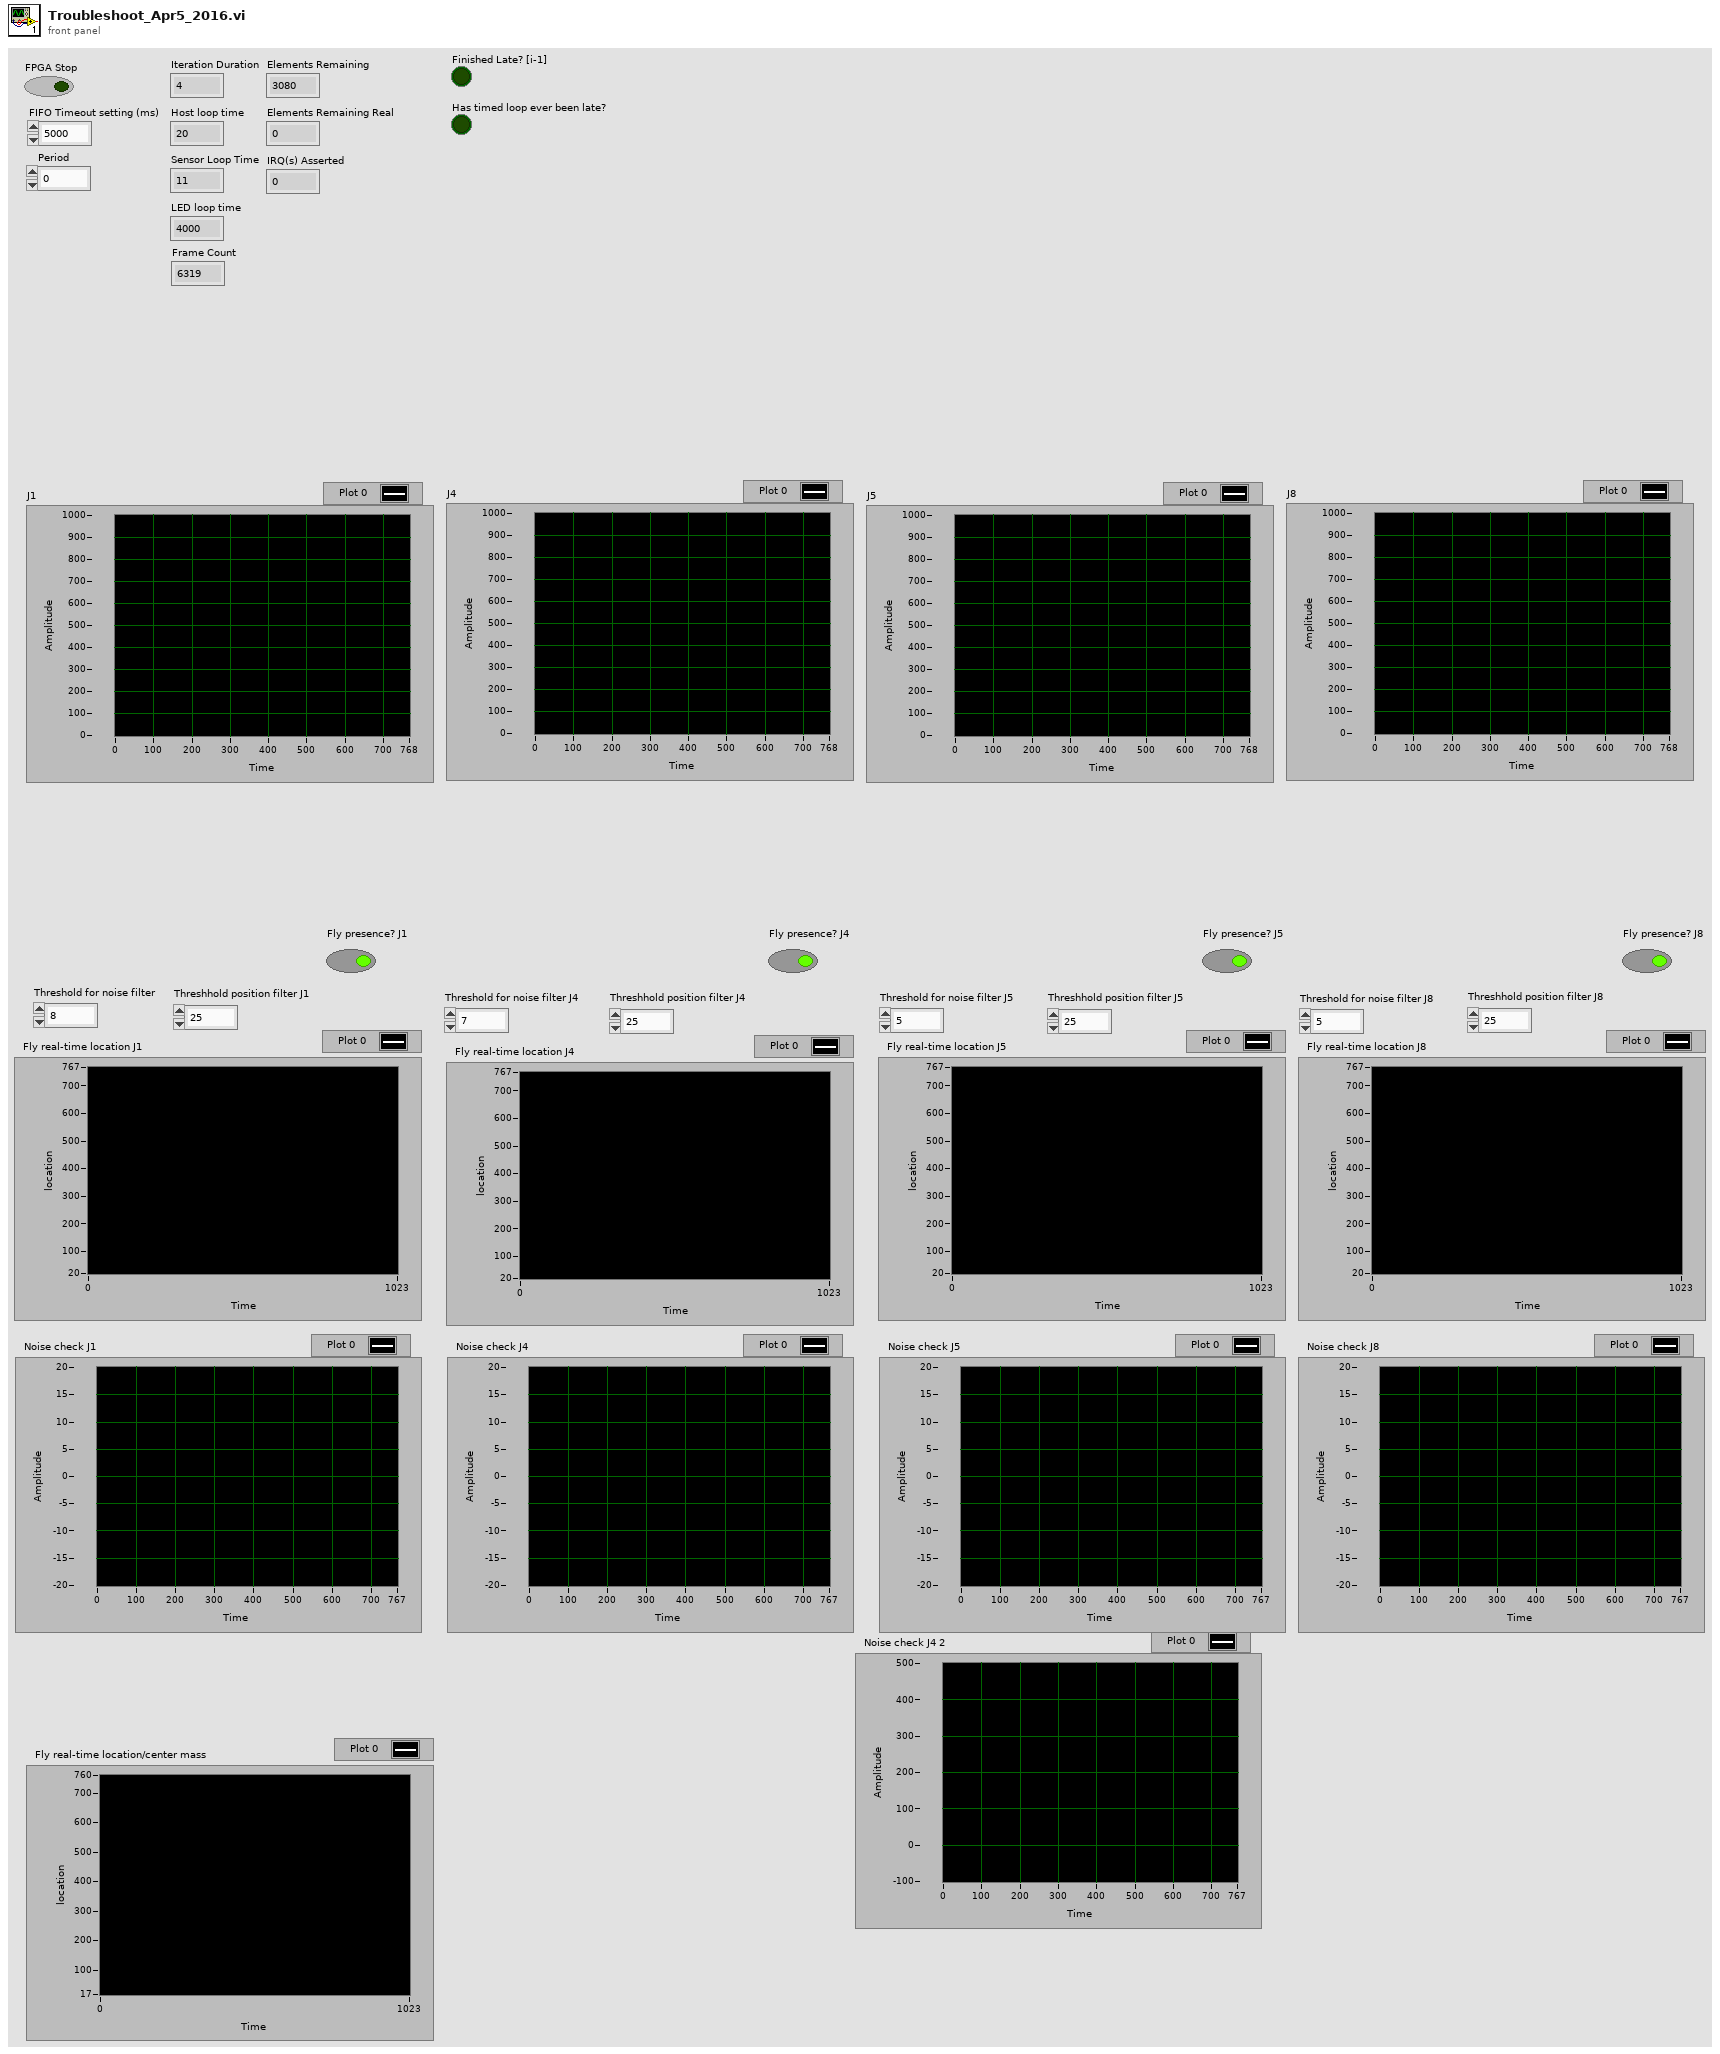
[diagram p1: front panel]
types:
  T1 = typedef "XDNodeRunTimeDep.lvlib/timing_clust.ctl" = cluster{"Expected End [f-1]":u64, "Actual End [f-1]":u64, "Finished Late? [f-1]":bool, "Expected End [i-1]":u64, "Actual End [i-1]":u64, "Finished Late? [i-1]":bool, "Expected Start [i]":u64, "Actual Start [i]":u64, "Expected Start [f]":u64, "Actual Start [f]":u64, "Source Name":string, "Structure Name":string, "Period":i64, "Deadline":i64, "Offset":i64, "Start":i64, "Priority":i32, "Timeout":i32, "Mode":T2, "Wakeup Reason":T3, "Error":errorcluster, "Source Type":string, "Secondary Source Type":string, "Global End Time":u64, "Global Start Time":u64, "Frame Duration":u64, "Iteration Duration":u64, "Assigned CPU":i32, "I/O Scan Engine Mode":u32}
  T2 = typedef "XDNodeRunTimeDep.lvlib/nitl_modes.ctl" = enum32{"No Change", "Process missed periods, maintain original phase", "Discard missed periods, maintain original phase", "Process missed periods, ignore original phase", "Discard missed periods, ignore original phase"}
  T3 = typedef "XDNodeRunTimeDep.lvlib/wakeup.ctl" = enum32{"Normal", "Aborted", "Asynchronous wakeup", "Timing source error", "Timed loop error", "Timeout"}
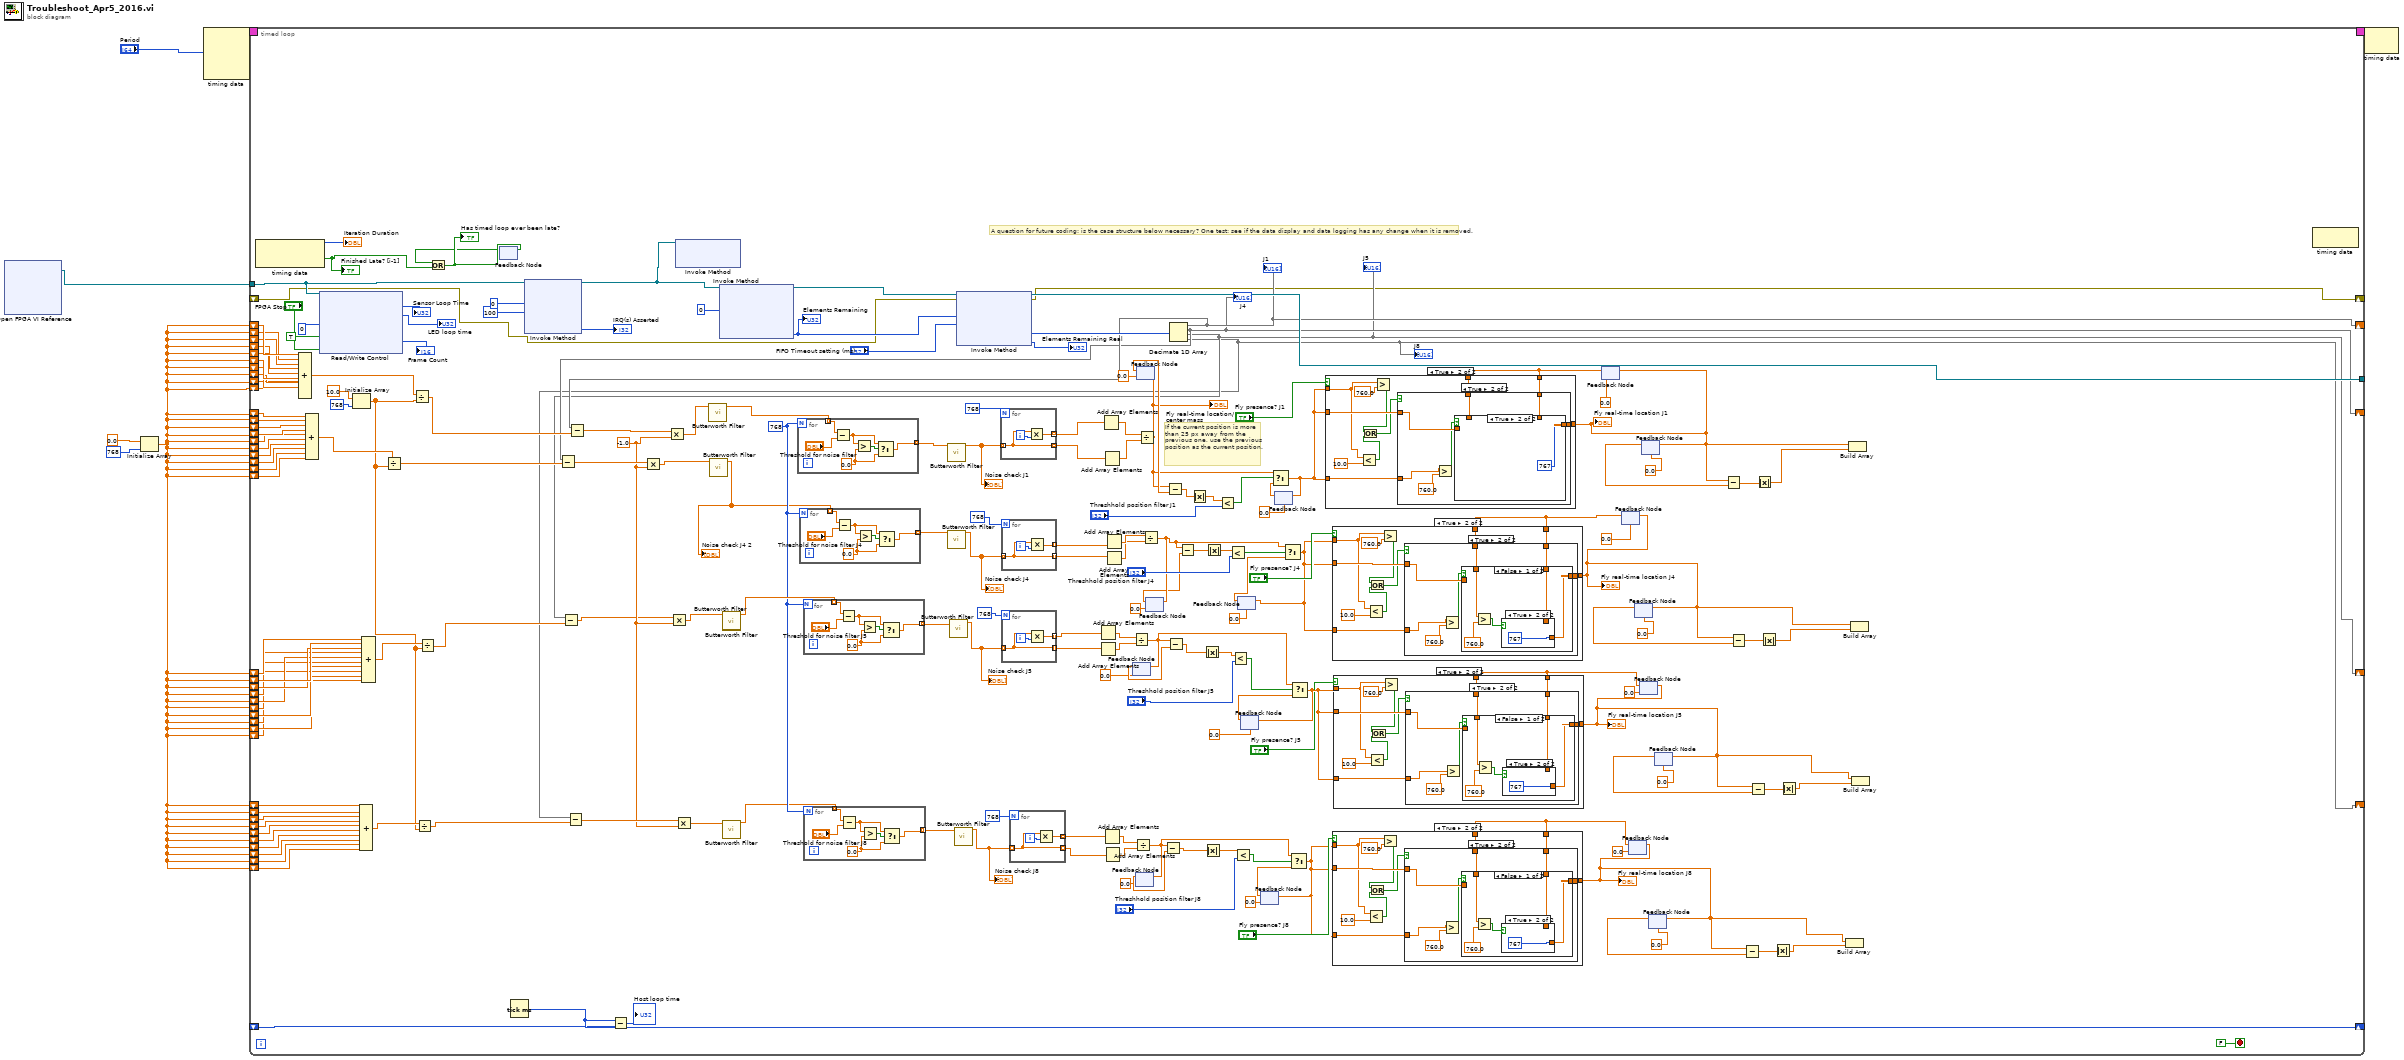
[diagram p0: block diagram]
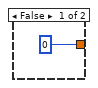
[diagram p2: hidden frame]
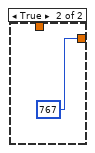
[diagram p5: hidden frame]
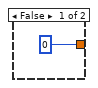
[diagram p6: hidden frame]
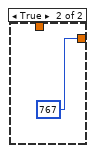
[diagram p9: hidden frame]
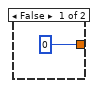
[diagram p10: hidden frame]
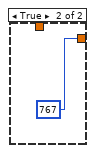
[diagram p13: hidden frame]
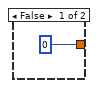
[diagram p14: hidden frame]
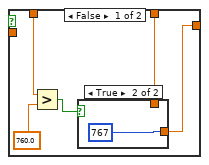
[diagram p16: hidden frame]
diagram:
  n1 = xnode "Open FPGA VI Reference"() -> ("FPGA VI Reference Out"=w5:refnum<k20>)  [unwired: 2 in, 1 out]
  n2 = Initialize Array(0.0 ("element"), 768 ("dimension size")) -> (w2:dbl[])
  n3 = node-c288("Period") -> (w7:T1)  [unwired: 3 in]
  n4 = timed-loop {
    tunnel: w5 -> [w186]
    shift-right: [w202] -> _
    shift-left: _ -> [w201]
    timing: w7 -> [_]
    timing-out: [_] -> w6
    tunnel: [w187] -> _
    shift-right: [w32] -> _
    shift-left: w2 -> [w164]
    shift-left: w2 -> [w163]
    shift-left: w2 -> [w162]
    shift-left: w2 -> [w161]
    shift-left: w2 -> [w160]
    shift-left: w2 -> [w159]
    shift-left: w2 -> [w158]
    shift-left: w2 -> [w157]
    shift-left: w2 -> [w156]
    shift-left: w2 -> [w155]
    shift-right: [w30] -> _
    shift-left: w2 -> [w89]
    shift-left: w2 -> [w88]
    shift-left: w2 -> [w87]
    shift-left: w2 -> [w86]
    shift-left: w2 -> [w85]
    shift-left: w2 -> [w84]
    shift-left: w2 -> [w83]
    shift-left: w2 -> [w82]
    shift-left: w2 -> [w81]
    shift-left: w2 -> [w80]
    shift-right: [w31] -> _
    shift-left: w2 -> [w102]
    shift-left: w2 -> [w101]
    shift-left: w2 -> [w100]
    shift-left: w2 -> [w99]
    shift-left: w2 -> [w98]
    shift-left: w2 -> [w97]
    shift-left: w2 -> [w96]
    shift-left: w2 -> [w95]
    shift-left: w2 -> [w94]
    shift-left: w2 -> [w93]
    shift-right: [w33] -> _
    shift-left: w2 -> [w49]
    shift-left: w2 -> [w48]
    shift-left: w2 -> [w47]
    shift-left: w2 -> [w46]
    shift-left: w2 -> [w45]
    shift-left: w2 -> [w44]
    shift-left: w2 -> [w43]
    shift-left: w2 -> [w42]
    shift-left: w2 -> [w41]
    shift-left: w2 -> [w40]
    shift-right: [w9] -> _
    shift-left: _ -> [w8]
    stop <- FALSE stop-if-true
    w74 = 768
    w76 = -1.0 ("y")
    # "If the current position is more than 25 px away from the previous one, use the previous position as the current position."
    # "A question for future coding: is the case structure below necessary? One test: see if the data display and data logging has any change when it is removed."
    n5 = node-c288() -> (→"Iteration Duration":i64, w180:bool)  [unwired: 1 in]
    "Finished Late? [i-1]" <- w180
    n6 = Compound Arithmetic op=ADD(w49, w48, w47, w46, w45, w44, w43, w42, w41, w40) -> (w39:dbl[])
    n7 = Compound Arithmetic op=ADD(w164, w163, w162, w161, w160, w159, w158, w157, w156, w155) -> (w154:dbl[])
    n8 = xnode "Read/Write Control"("FPGA VI Reference In"=w186, "IRQ Bit (0-31)"=u8 0 ("IRQ Bit (0-31) J1"), "Wait Until IRQ Cleared?"=TRUE ("Wait Until IRQ Cleared? J1"), "FPGA Stop"="FPGA Stop") -> ("Sensor Loop Time"=→"Sensor Loop Time":u32, "LED loop time"=→"LED loop time":u32, "Frame Count"=→"Frame Count":i16)  [unwired: 1 in, 2 out]
    n9 = Initialize Array(10.0 ("element"), 768 ("dimension size")) -> (w53:dbl[])
    n10 = Compound Arithmetic op=ADD(w89, w88, w87, w86, w85, w84, w83, w82, w81, w80) -> (w79:dbl[])
    n11 = Compound Arithmetic op=ADD(w102, w101, w100, w99, w98, w97, w96, w95, w94, w93) -> (w139:dbl[])
    n12 = Divide(x=w154, y=w53) -> (x/y=w153:dbl[])
    n13 = Divide(x=w39, y=w53) -> (x/y=w52:dbl[])
    n14 = Divide(x=w79, y=w53) -> (x/y=w78:dbl[])
    n15 = Divide(x=w139, y=w53) -> (x/y=w50:dbl[])
    n16 = feedback #1() -> (w184:bool)  [unwired: 1 in]
    n17 = Or(x=w184, y=w180) -> (x .or. y?=w185:bool)
    "Has timed loop ever been late?" <- w185
    n18 = feedback-in #1(w185) -> ()
    n19 = Tick Count (ms)() -> (millisecond timer value=w202:u32)
    n20 = xnode "Invoke Method"("FPGA VI Reference In"=w186, "IRQ Number(s)"=0, "Timeout (ms)"=100) -> ("FPGA VI Reference Out"=w178:refnum<k20>, "IRQ(s) Asserted"=→"IRQ(s) Asserted":i32)  [unwired: 1 in, 2 out]
    n21 = Subtract(x=w202, y=w201) -> (x-y=→"Host loop time":u32)
    n22 = xnode "Invoke Method"("FPGA VI Reference In"=w178) -> ()  [unwired: 2 in, 2 out]
    n23 = xnode "Invoke Method"("FPGA VI Reference In"=w178, "Number of Elements"=u32 0) -> ("FPGA VI Reference Out"=w189:refnum<k20>, "Elements Remaining"=w188:u32)  [unwired: 2 in, 2 out]
    "Elements Remaining" <- w188
    n24 = call-poly <vilib>:"Butterworth Filter.vi"() -> ()  [unwired: 8 in, 2 out]
    n25 = xnode "Invoke Method"("FPGA VI Reference In"=w189, "error in"=w8, "Number of Elements"=w188, "Timeout (ms)"="FIFO Timeout setting (ms)") -> ("FPGA VI Reference Out"=w187:refnum<k20>, "error out"=w9:errorcluster, "Data"=w190:u16[], "Elements Remaining"=→"Elements Remaining Real":u32)
    n26 = feedback #2(0.0) -> (w116:dbl)
    n27 = feedback #3(0.0) -> (w63:dbl)
    n28 = feedback #4(0.0) -> (w129:dbl)
    n29 = feedback #5(0.0) -> (w124:dbl)
    n30 = Decimate 1D Array(w190) -> (w33:u16[], w32:u16[], w31:u16[], w30:u16[])
    "J1" <- w33
    "J4" <- w32
    "J8" <- w30
    "J5" <- w31
    n31 = Subtract(x=w32, y=w153) -> (x-y=w152:dbl[])
    n32 = Subtract(x=w31, y=w50) -> (x-y=w51:dbl[])
    n33 = Subtract(x=w30, y=w78) -> (x-y=w77:dbl[])
    n34 = Subtract(x=w33, y=w52) -> (x-y=w91:dbl[])
    n35 = Multiply(x=w152, y=w76) -> (x*y=w151:dbl[])
    n36 = Multiply(x=w91, y=w76) -> (x*y=w170:dbl[])
    n37 = Multiply(x=w51, y=w76) -> (x*y=w103:dbl[])
    n38 = Multiply(x=w77, y=w76) -> (x*y=w75:dbl[])
    n39 = call-poly <vilib>:"Butterworth Filter.vi"("X"=w170) -> ("Filtered X"=w90:dbl[])  [unwired: 7 in, 1 out]
    n40 = call-poly <vilib>:"Butterworth Filter.vi"("X"=w151) -> ("Filtered X"=w34:dbl[])  [unwired: 7 in, 1 out]
    "Noise check J4 2" <- w34
    n41 = call-poly <vilib>:"Butterworth Filter.vi"("X"=w103) -> ("Filtered X"=w92:dbl[])  [unwired: 7 in, 1 out]
    n42 = call-poly <vilib>:"Butterworth Filter.vi"("X"=w75) -> ("Filtered X"=w73:dbl[])  [unwired: 7 in, 1 out]
    n43 = for {
      N: w74 -> [_]
      tunnel: w90 -> [w352] mode=indexing
      tunnel: [w348] -> w176 mode=indexing
      w349 = 0.0 ("y")
      n44 = Subtract(x=w352, y="Threshold for noise filter") -> (x-y=w350:dbl)
      n45 = Greater?(x=w350, y=w349) -> (0:w351:bool)
      n46 = Select(t=w350, s=w351, f=w349) -> (s? t:f=w348:dbl)
    }
    n47 = for {
      N: w74 -> [_]
      tunnel: w34 -> [w315] mode=indexing
      tunnel: [w311] -> w150 mode=indexing
      w312 = 0.0 ("y")
      n48 = Subtract(x=w315, y="Threshold for noise filter J4") -> (x-y=w313:dbl)
      n49 = Greater?(x=w313, y=w312) -> (0:w314:bool)
      n50 = Select(t=w313, s=w314, f=w312) -> (s? t:f=w311:dbl)
    }
    n51 = for {
      N: w74 -> [_]
      tunnel: w92 -> [w278] mode=indexing
      tunnel: [w274] -> w123 mode=indexing
      w275 = 0.0 ("y")
      n52 = Subtract(x=w278, y="Threshold for noise filter J5") -> (x-y=w276:dbl)
      n53 = Greater?(x=w276, y=w275) -> (0:w277:bool)
      n54 = Select(t=w276, s=w277, f=w275) -> (s? t:f=w274:dbl)
    }
    n55 = for {
      N: w74 -> [_]
      tunnel: w73 -> [w241] mode=indexing
      tunnel: [w237] -> w72 mode=indexing
      w238 = 0.0 ("y")
      n56 = Subtract(x=w241, y="Threshold for noise filter J8") -> (x-y=w239:dbl)
      n57 = Greater?(x=w239, y=w238) -> (0:w240:bool)
      n58 = Select(t=w239, s=w240, f=w238) -> (s? t:f=w237:dbl)
    }
    n59 = call-poly <vilib>:"Butterworth Filter.vi"("X"=w176) -> ("Filtered X"=w38:dbl[])  [unwired: 7 in, 1 out]
    "Noise check J1" <- w38
    n60 = call-poly <vilib>:"Butterworth Filter.vi"("X"=w150) -> ("Filtered X"=w37:dbl[])  [unwired: 7 in, 1 out]
    "Noise check J4" <- w37
    n61 = call-poly <vilib>:"Butterworth Filter.vi"("X"=w123) -> ("Filtered X"=w36:dbl[])  [unwired: 7 in, 1 out]
    "Noise check J5" <- w36
    n62 = call-poly <vilib>:"Butterworth Filter.vi"("X"=w72) -> ("Filtered X"=w35:dbl[])  [unwired: 7 in, 1 out]
    "Noise check J8" <- w35
    n63 = for {
      N: 768 -> [_]
      tunnel: w38 -> [w344] mode=indexing
      tunnel: [w345] -> w174 mode=indexing
      tunnel: [w344] -> w173 mode=indexing
      i -> [w346]
      n64 = Multiply(x=w344, y=w346) -> (x*y=w345:dbl)
    }
    n65 = for {
      N: 768 -> [_]
      tunnel: w37 -> [w307] mode=indexing
      tunnel: [w308] -> w147 mode=indexing
      tunnel: [w307] -> w148 mode=indexing
      i -> [w309]
      n66 = Multiply(x=w307, y=w309) -> (x*y=w308:dbl)
    }
    n67 = for {
      N: 768 -> [_]
      tunnel: w36 -> [w270] mode=indexing
      tunnel: [w271] -> w121 mode=indexing
      tunnel: [w270] -> w120 mode=indexing
      i -> [w272]
      n68 = Multiply(x=w270, y=w272) -> (x*y=w271:dbl)
    }
    n69 = for {
      N: 768 -> [_]
      tunnel: w35 -> [w233] mode=indexing
      tunnel: [w234] -> w70 mode=indexing
      tunnel: [w233] -> w69 mode=indexing
      i -> [w235]
      n70 = Multiply(x=w233, y=w235) -> (x*y=w234:dbl)
    }
    n71 = Add Array Elements(numeric array=w121) -> (sum=w119:dbl)
    n72 = Add Array Elements(numeric array=w120) -> (sum=w118:dbl)
    n73 = Add Array Elements(numeric array=w174) -> (sum=w172:dbl)
    n74 = Add Array Elements(numeric array=w173) -> (sum=w171:dbl)
    n75 = Add Array Elements(numeric array=w70) -> (sum=w68:dbl)
    n76 = Add Array Elements(numeric array=w69) -> (sum=w67:dbl)
    n77 = Add Array Elements(numeric array=w147) -> (sum=w146:dbl)
    n78 = Add Array Elements(numeric array=w148) -> (sum=w145:dbl)
    n79 = Divide(x=w119, y=w118) -> (x/y=w104:dbl)
    n80 = feedback-in #2(w104) -> ()
    n81 = Divide(x=w68, y=w67) -> (x/y=w58:dbl)
    n82 = feedback-in #3(w58) -> ()
    n83 = Divide(x=w172, y=w171) -> (x/y=w128:dbl)
    "Fly real-time location/center mass" <- w128
    n84 = feedback-in #4(w128) -> ()
    n85 = Divide(x=w146, y=w145) -> (x/y=w126:dbl)
    n86 = feedback-in #5(w126) -> ()
    n87 = Subtract(x=w58, y=w63) -> (x-y=w66:dbl)
    n88 = Subtract(x=w128, y=w129) -> (x-y=w168:dbl)
    n89 = Subtract(x=w104, y=w116) -> (x-y=w115:dbl)
    n90 = Subtract(x=w126, y=w124) -> (x-y=w144:dbl)
    n91 = Absolute Value(x=w168) -> (abs(x)=w167:dbl)
    n92 = Absolute Value(x=w115) -> (abs(x)=w114:dbl)
    n93 = Absolute Value(x=w66) -> (abs(x)=w65:dbl)
    n94 = Absolute Value(x=w144) -> (abs(x)=w143:dbl)
    n95 = Less?(x=w167, y="Threshhold position filter J1") -> (x < y?=w165:bool)
    n96 = Less?(x=w143, y="Threshhold position filter J4") -> (x < y?=w141:bool)
    n97 = Less?(x=w114, y="Threshhold position filter J5") -> (x < y?=w110:bool)
    n98 = Less?(x=w65, y="Threshhold position filter J8") -> (x < y?=w64:bool)
    n99 = feedback #6(0.0) -> (w134:dbl)
    n100 = feedback #7(0.0) -> (w111:dbl)
    n101 = feedback #8(0.0) -> (w60:dbl)
    n102 = feedback #9(0.0) -> (w131:dbl)
    n103 = Select(t=w128, s=w165, f=w131) -> (s? t:f=w132:dbl)
    n104 = feedback-in #9(w132) -> ()
    n105 = Select(t=w126, s=w141, f=w134) -> (s? t:f=w135:dbl)
    n106 = feedback-in #6(w135) -> ()
    n107 = Select(t=w58, s=w64, f=w60) -> (s? t:f=w56:dbl)
    n108 = feedback-in #8(w56) -> ()
    n109 = Select(t=w104, s=w110, f=w111) -> (s? t:f=w108:dbl)
    n110 = feedback-in #7(w108) -> ()
    n111 = feedback #10(0.0) -> (w138:dbl)
    n112 = case shown="True" "Fly presence? J1" {
      tunnel: w132 -> [_ w327]
      tunnel: [0 w326] -> w27
      tunnel: w132 -> [_ w320]
      tunnel: w132 -> [_ w319]
      tunnel: w138 -> [_ w318]
      tunnel: w138 -> [_ w317]
      frame False {
      }
      frame True {
        n113 = Less?(x=w320, y=10.0) -> (x < y?=w323:bool)
        n114 = Greater?(x=w320, y=760.0) -> (0:w321:bool)
        n115 = Or(x=w321, y=w323) -> (x .or. y?=w325:bool)
        n116 = case shown="True" w325 {
          tunnel: w327 -> [w328 w334]
          tunnel: [w328 w335] -> w326
          tunnel: w319 -> [_ w329]
          tunnel: w318 -> [_ w332]
          tunnel: w317 -> [_ w330]
          frame False {
          }
          frame True {
            n117 = Greater?(x=w329, y=760.0) -> (0:w331:bool)
            n118 = case shown="True" w331 {
              tunnel: [w338 767] -> w335
              tunnel: w334 -> [_ _]
              tunnel: w332 -> [w340 _]
              tunnel: w330 -> [w336 _]
              frame False {
                n119 = Greater?(x=w340, y=760.0) -> (0:w337:bool)
                n120 = case shown="True" w337 {
                  tunnel: [w341 767] -> w338
                  tunnel: w336 -> [w341 _]
                  frame False {
                  }
                  frame True {
                  }
                }
              }
              frame True {
              }
            }
          }
        }
      }
    }
    "Fly real-time location J1" <- w27
    n121 = feedback-in #10(w27) -> ()
    n122 = feedback #11(0.0) -> (w117:dbl)
    n123 = case shown="True" "Fly presence? J4" {
      tunnel: w135 -> [_ w290]
      tunnel: [0 w289] -> w20
      tunnel: w135 -> [_ w283]
      tunnel: w135 -> [_ w282]
      tunnel: w117 -> [_ w281]
      tunnel: w117 -> [_ w280]
      frame False {
      }
      frame True {
        n124 = Less?(x=w283, y=10.0) -> (x < y?=w286:bool)
        n125 = Greater?(x=w283, y=760.0) -> (0:w284:bool)
        n126 = Or(x=w284, y=w286) -> (x .or. y?=w288:bool)
        n127 = case shown="True" w288 {
          tunnel: w290 -> [w291 w297]
          tunnel: [w291 w298] -> w289
          tunnel: w282 -> [_ w292]
          tunnel: w281 -> [_ w295]
          tunnel: w280 -> [_ w293]
          frame False {
          }
          frame True {
            n128 = Greater?(x=w292, y=760.0) -> (0:w294:bool)
            n129 = case shown="False" w294 {
              tunnel: [w301 767] -> w298
              tunnel: w297 -> [_ _]
              tunnel: w295 -> [w303 _]
              tunnel: w293 -> [w299 _]
              frame False {
                n130 = Greater?(x=w303, y=760.0) -> (0:w300:bool)
                n131 = case shown="True" w300 {
                  tunnel: [w304 767] -> w301
                  tunnel: w299 -> [w304 _]
                  frame False {
                  }
                  frame True {
                  }
                }
              }
              frame True {
              }
            }
          }
        }
      }
    }
    "Fly real-time location J4" <- w20
    n132 = feedback-in #11(w20) -> ()
    n133 = feedback #12(0.0) -> (w55:dbl)
    n134 = case shown="True" "Fly presence? J8" {
      tunnel: w56 -> [_ w216]
      tunnel: [0 w215] -> w10
      tunnel: w56 -> [_ w209]
      tunnel: w56 -> [_ w208]
      tunnel: w55 -> [_ w207]
      tunnel: w55 -> [_ w206]
      frame False {
      }
      frame True {
        n135 = Less?(x=w209, y=10.0) -> (x < y?=w212:bool)
        n136 = Greater?(x=w209, y=760.0) -> (0:w210:bool)
        n137 = Or(x=w210, y=w212) -> (x .or. y?=w214:bool)
        n138 = case shown="True" w214 {
          tunnel: w216 -> [w217 w223]
          tunnel: [w217 w224] -> w215
          tunnel: w208 -> [_ w218]
          tunnel: w207 -> [_ w221]
          tunnel: w206 -> [_ w219]
          frame False {
          }
          frame True {
            n139 = Greater?(x=w218, y=760.0) -> (0:w220:bool)
            n140 = case shown="False" w220 {
              tunnel: [w227 767] -> w224
              tunnel: w223 -> [_ _]
              tunnel: w221 -> [w229 _]
              tunnel: w219 -> [w225 _]
              frame False {
                n141 = Greater?(x=w229, y=760.0) -> (0:w226:bool)
                n142 = case shown="True" w226 {
                  tunnel: [w230 767] -> w227
                  tunnel: w225 -> [w230 _]
                  frame False {
                  }
                  frame True {
                  }
                }
              }
              frame True {
              }
            }
          }
        }
      }
    }
    "Fly real-time location J8" <- w10
    n143 = feedback-in #12(w10) -> ()
    n144 = feedback #13(0.0) -> (w22:dbl)
    n145 = feedback-in #13(w20) -> ()
    n146 = feedback #14(0.0) -> (w107:dbl)
    n147 = case shown="True" "Fly presence? J5" {
      tunnel: w108 -> [_ w253]
      tunnel: [0 w252] -> w16
      tunnel: w108 -> [_ w246]
      tunnel: w108 -> [_ w245]
      tunnel: w107 -> [_ w244]
      tunnel: w107 -> [_ w243]
      frame False {
      }
      frame True {
        n148 = Less?(x=w246, y=10.0) -> (x < y?=w249:bool)
        n149 = Greater?(x=w246, y=760.0) -> (0:w247:bool)
        n150 = Or(x=w247, y=w249) -> (x .or. y?=w251:bool)
        n151 = case shown="True" w251 {
          tunnel: w253 -> [w254 w260]
          tunnel: [w254 w261] -> w252
          tunnel: w245 -> [_ w255]
          tunnel: w244 -> [_ w258]
          tunnel: w243 -> [_ w256]
          frame False {
          }
          frame True {
            n152 = Greater?(x=w255, y=760.0) -> (0:w257:bool)
            n153 = case shown="False" w257 {
              tunnel: [w264 767] -> w261
              tunnel: w260 -> [_ _]
              tunnel: w258 -> [w266 _]
              tunnel: w256 -> [w262 _]
              frame False {
                n154 = Greater?(x=w266, y=760.0) -> (0:w263:bool)
                n155 = case shown="True" w263 {
                  tunnel: [w267 767] -> w264
                  tunnel: w262 -> [w267 _]
                  frame False {
                  }
                  frame True {
                  }
                }
              }
              frame True {
              }
            }
          }
        }
      }
    }
    "Fly real-time location J5" <- w16
    n156 = feedback-in #14(w16) -> ()
    n157 = feedback-in #15(w27) -> ()
    n158 = feedback #15(0.0) -> (w29:dbl)
    n159 = feedback #16(0.0) -> (w12:dbl)
    n160 = feedback-in #16(w10) -> ()
    n161 = feedback #17(0.0) -> (w17:dbl)
    n162 = feedback-in #17(w16) -> ()
    n163 = Subtract(x=w27, y=w29) -> (x-y=w26:dbl)
    n164 = Subtract(x=w20, y=w22) -> (x-y=w23:dbl)
    n165 = Subtract(x=w10, y=w12) -> (x-y=w13:dbl)
    n166 = Subtract(x=w16, y=w17) -> (x-y=w18:dbl)
    n167 = Absolute Value(x=w26) -> (abs(x)=w25:dbl)
    n168 = Absolute Value(x=w23) -> (abs(x)=w21:dbl)
    n169 = Absolute Value(x=w13) -> (abs(x)=w11:dbl)
    n170 = Absolute Value(x=w18) -> (abs(x)=w15:dbl)
    n171 = Build Array(w10, w11) -> ()  [unwired: 1 out]
    n172 = Build Array(w27, w25) -> ()  [unwired: 1 out]
    n173 = Build Array(w20, w21) -> ()  [unwired: 1 out]
    n174 = Build Array(w16, w15) -> ()  [unwired: 1 out]
    n175 = node-c288() -> ()  [unwired: 1 in, 1 out]
  }
  n176 = node-c288(w6) -> ()  [unwired: 1 out]
